vi "UHR-Fleezers Control (fpga) - Leonardo 04-2018 V4.vi"() -> ()   [LabVIEW 2013]
doc: "UHR-Fleezers Instrument Control Code (fpga)"
uses:
  <vilib>/Platform/TimedLoop/XDataNode/timing_clust.ctl
  <vilib>/Platform/TimedLoop/XDataNode/nitl_modes.ctl
  <vilib>/Platform/TimedLoop/XDataNode/wakeup.ctl
  <vilib>/rvi/eio/common/nirviEmuTemplateMethod_errors.vi
  <vilib>/rvi/Emulation/niFpgaSctlEmulationGetInTimedLoop.vi
  <vilib>/rvi/Emulation/niFpgaEmulationReportErrorSimple.vi
  <vilib>/rvi/Emulation/niFpgaGetClockAttributes.vi
  <vilib>/rvi/Emulation/niFpgaCriticalErrorInLSC.vi
  <vilib>/rvi/FIFO/Fifo_Resource/nirvififoEmulationReadFpgaImpl.vi
  <vilib>/rvi/DataTransferAndStorage/Container/Common/niFpgaContainerGetUniqueNameForEmu.vi
  <vilib>/rvi/DataTransferAndStorage/Container/Common/niFpgaContainerExecOnDevCompGetState.vi
  <vilib>/rvi/interface/RandomDataEmulation/nirviRandomDataFPGAFIFO.vi
  <vilib>/rvi/interface/RandomDataEmulation/niFpgaRandomDataHandleErrors.vi
  <vilib>/rvi/eio/common/nirviEmuReportErrorAndStop.vi
  <vilib>/rvi/Emulation/niFpgaProcessEmulError.vi
  <vilib>/rvi/FIFO/Fifo_Resource/nirvififoEmulationWriteFpgaImpl.vi
  <vilib>/Platform/TimedLoop/XDataNode/XDataNode.xnode
  <vilib>/eio/EIOMethodNode/EIOMethodNode.xnode
  <vilib>/eio/EIONode/EIONode.xnode
  <vilib>/rvi/DataTransferAndStorage/Container/XNode/niFpgaContainer.xnode
  <vilib>/rvi/FIFO/Fifo_Resource/nirvififoEmulationRead.vi
  <vilib>/rvi/FIFO/Fifo_Resource/niFpgaFifoEmulationRefIn.vi
  <vilib>/rvi/interface/RandomDataEmulation/nirviRandomDataFpgaReadWriteTemplate.vi
  <vilib>/rvi/FIFO/Fifo_Resource/nirvififoEmulationWrite.vi
  <vilib>/addons/control/pid/fpga.llb/XNode/niFpgaPID.xnode
  <vilib>/Platform/TimedLoop/XDataNode/XDNodeRunTimeDep.lvlib
  <vilib>/rvi/Memory/Memory_Emulation/niFpgaMemoryEmulationRefIn.vi
panel:
  in  "Tab Control 2":T1(tab)
  out "BD1 amplitude 1 out":u16
  out "BD1 amplitude 2 out":u16
  in  "FB output range":cluster{"output low":i16, "output high":i16}={"output low"=0, "output high"=3000}
  in  "FB Gains":T2={"proportional gain (Kc)"=10, "integral gain (Kc*Ts/Ti)"=5, "derivative gain (Kc*Td/Ts)"=0}
  in  "RF synth green feedback max":i16=4000
  in  "RD":bool=TRUE
  in  "Swap F1 and F2":bool
  in  "Scan BD":bool
  in  "Start scan":bool
  in  "OSK Bd 1":bool
  in  "Reset Bd 1":bool
  in  "PMODE":bool=TRUE
  in  "Number Interlace Cycles":u8=2 min=1 max=3
  in  "Interlace Off Parameters":u8=1 min=1 max=3
  in  "Interlace ON/OFF":bool
  out "DIO Relative phase":i16
  in  "Phase count adjustment (DIO)":i16
  in  "+ phase (DIO)":bool
  out "DIO Late Counter":u8
  in  "DIO count 1 (ticks)":u16=400
  in  "DIO count 2 (ticks)":u16=400
  in  "DIO count 3 (ticks)":u16=400
  out "AI2 Y Sum Set 2":i16
  out "AI2 Y Sum Set 1":i16
  in  "FB Setpoint Set 1":i16 min=0 step=1
  in  "FB Reset Set 1":bool
  in  "FB On/Off Set 1":bool
  in  "FB Reset Set 2":bool
  in  "FB On/Off Set 2":bool
  in  "FB Setpoint Set 2":i16 min=0 step=1
  in  "Amp switch delay":u8=5
  in  "RF synth bd controls green":bool
  in  "Phase Trap 2":fxp<+,14,14>
  in  "Phase Trap 1":fxp<+,14,14>
  in  "Phase offset method":u8
  in  "BD 2 Amplitude 1":u16
  in  "BD 1 Amplitude 1":u16
  in  "BD 2 Frequency 1":u64
  in  "BD 1 Frequency 1":u64
  in  "BD 2 Amplitude 2":u16
  in  "BD 1 Amplitude 2":u16
  in  "BD 2 Frequency 2":u64
  in  "BD 1 Frequency 2":u64
  in  "BD 2 Amplitude 3":u16
  in  "BD 1 Amplitude 3":u16
  in  "BD 2 Frequency 3":u64
  in  "BD 1 Frequency 3":u64
  in  "BD 2 Delay (Ticks)":u8 caption="Count(Ticks)"
  in  "Next trap write delay (ticks)":u8 caption="Count(Ticks)"
  out "Random phase generated":fxp<+,14,14>
  in  "RF phase reset before cycles":bool
  in  "Trap 1 osc enable":bool
  in  "N trap osc periods":i16
  in  "Trap osc period (pts)":i16
  in  "Osc traps":bool
  in  "Initiate trap osc":bool
  in  "Ready Write":bool
  in  "Data":i64
  in  "Address 2":u32
  in  "Osc trap cont.":bool
  in  "Trap 2 osc enable":bool
  out "green FB running":bool
  in  "APD 2 AO scale factor":i16=1
  in  "BD 1 Delay (ticks)":u8
  in  "Tab Control":T3(tab)=enum."MCL trap control"
  in  "Set 3":bool
  in  "Set 2":bool=TRUE
  in  "Set 1":bool=TRUE
  in  "Trap Pos to FIFO":bool
  in  "N of AI1 Int Acq Sets":i16=2 min=1 max=3 step=1
  out "AI Late Counter":u8
  in  "ai count":u16=400
  in  "+ phase":bool
  in  "Phase count adjustment":i16
  out "Relative phase":i16
  in  "AI to FIFO":bool
  out "BD1 Frequency Out 1":u64
  out "BD1 Frequency Out 2":u64
  out "Trap Pos FIFO Timeout":u16
  out "Trap AI FIFO Timeout":u16
  in  "Trap FIFO Set Timeout":i32
  in  "Scan freq.  increment":i64
  in  "Scan steps":u64
  in  "Number of scans":u16
  in  "Cycles per step":u64
  in  "Raster setpoint":fxp<+/-,16,1>
  in  "Raster to target force":bool
  out "Actual Scan freq":u64
  in  "Cont. Scan":bool
  out "Scan I":u64
  in  "Abort scan":bool
  out "Scanning":bool
  in  "FB Min frequency":u64
  in  "FB Max Frequency":u64
  in  "Dynamic Force FB (Ronen)":bool
  in  "Trap pos. FB Range":T4={"FB2 output low"=-1.0, "FB2 output high"=0.999969482421875}
  in  "Trap Pos. FB Gains":T5={"proportional gain (Kc)"=0.999969482421875, "integral gain (Kc*Ts/Ti)"=0.999969482421875, "derivative gain (Kc*Td/Ts)"=0.0}
  in  "B factor":fxp<+/-,32,16>
  in  "Negate Diff?":bool
  in  "Diff FB Measurement?":bool
  in  "FB Trig Integrate":u32=1
  out "TTrig?":bool
  in  "TTrig Negate Pos":bool=TRUE
  out "Trap Pos FB Int Signal":fxp<+/-,24,9> format="%.18g"
  out "Trap Pos FB Int-Norm Signal":fxp<+/-,16,1> format="%.16g"
  in  "FPGA TTrig Thresh":i64
  in  "FPGA Trap Trig":bool
  out "Trap Pos FB Action":i64
  in  "Trap Pos. FB Offset Factor":i64
  in  "Trap Pos. FB Mult Factor":i64=2
  in  "Trap Pos. FB Reset":bool
  in  "Trap Pos FB Monitor T1 or T2":bool
  in  "AI1 X Scale":u16
  in  "Trap Pos FB Int Count":u16=100
  in  "Trap Pos FB Negate Action":bool
  out "AI1 X Set 2":fxp<+/-,16,1>
  out "AI1 X Set 1":fxp<+/-,16,1>
  in  "Trap Pos. FB SP":fxp<+/-,16,1>
  in  "Force feedback":bool
  out "TTrig Sig":i64
  out "TTrig Fin Thresh":i64
  in  "1D or 2D Scan?":bool
  in  "Abort scan (MCL)":bool
  in  "MCL Scan Axis":bool
  in  "Cont. Scan (MCL)":bool
  out "Scan I (MCL)":u64
  in  "Number of scans (MCL)":u16
  out "Scanning MCL":bool
  in  "Scan steps (MCL)":u64
  in  "Cycles per step (MCL)":u64
  in  "Scan freq.  increment (MCL)":i16
  in  "Start scan (MCL)":bool
  in  "AO2 (X)":i16
  in  "AO1 (Y)":i16
  out "MCL Late Counter":u8
  in  "MCL count":u32=800
  out "MCL Relative Phase":i16
  in  "Phase count adjustment (MCL)":i16
  in  "+ phase (MCL)":bool
  in  "Lifetime events to read blue":u16=100
  in  "Lifetime read blue fifo":bool
  out "lifetime events in fifo":u16
  out "APD2 int gate":bool
  in  "APD Gate Operating Mode":u8 max=2 step=1
  in  "Invert APD Gate":bool
  in  "APD Gate OFF Count":u16=100
  in  "APD Gate ON Count":u16=300
  out "APD 1 Gate Late Counter":u8
  out "APD 1 Gate Relative Phase":i16
  in  "Phase count adjustment (APD 1 Gate)":i16
  in  "+ phase (APD 1 Gate)":bool
  out "APD 2 Counts 0":u32
  out "APD 2 Counts 1":u32
  out "APD 1 Counts 0":u32
  out "APD 1 Counts 1":u32
  in  "Phase count adjustment (APD 2 Gate)":i16
  out "APD 2 Gate Late Counter":u8
  out "APD 2 Gate Relative Phase":i16
  in  "+ phase (APD 2 Gate)":bool
  out "APD 3 Counts 0":u32
  out "APD 3 Counts 1":u32
  out "APD 3 Gate Late Counter":u8
  in  "Phase count adjustment (APD 3 Gate)":i16
  out "APD 3 Gate Relative Phase":i16
  in  "+ phase (APD 3 Gate)":bool
  out "APD1 int gate":bool
  out "APD3 int gate":bool
  in  "Lifetime timeout APD1":u16=200
  in  "APD to FIFO":bool
  in  "APD Acq Rate Count":u32=20000000
  out "APD Acq Late Counter":u16
  out "APD Acq Relative Phase":i16
  in  "+ phase (APD Acq)":bool
  in  "Phase Count Adjustment (APD Acq)":i16
  in  "APD 1 AO scale factor":i16=1
  out "APD2 out state":bool
  out "APD1 out state":bool
  out "APD Acq Late?":bool
  in  "Number of OFF cycles":i16
  in  "Green long-scale interlacing":bool
  in  "D3 2":i16
  in  "I3 2":i16=5
  in  "P3 2":i16=10
  in  "Green FB Setpoint 2":i16=250 min=0 step=1
  in  "Green FB Reset 2":bool
  in  "Green Filter Flipper":bool
  in  "Green interlace OFF count":u16=100
  out "GI Relative phase":i16
  in  "Phase count adjustment (GI)":i16
  in  "+ phase (GI)":bool
  in  "Green interlace ON count":u16=300
  out "GI Late Counter":u8
  in  "Invert GI":bool
  in  "Operating Mode":u8 max=2 step=1
  in  "Current Out":u16=30000
  in  "Green int current ON count adj":u32=150
  in  "Green interlace OFF count 2":u32=900
  in  "Green interlace ON count 2":u32=300
  out "GI Late Counter 2":u16
  in  "Green FB Count":u32=1200
  in  "Phase count adjustment (GI) 2":i16=20
  in  "Green FB Setpoint":i16=250 min=0 step=1
  in  "Invert GI 2":bool
  out "GI Relative phase 2":i16
  in  "+ phase (GI) 2":bool
  in  "Phase count adjustment (Green FB)":i16=10
  out "Green Late Counter":u16
  out "Green FB Relative Phase":i16
  in  "+ phase (Green FB)":bool
  out "Green FB Signals":T6
  out "Green FB Sum":i16
  in  "Green FB Gains":T2={"proportional gain (Kc)"=10, "integral gain (Kc*Ts/Ti)"=5, "derivative gain (Kc*Td/Ts)"=0}
  in  "Green FB On/Off":bool
  in  "Green FB Reset":bool
  out "Green FB Late?":bool
  out "GI Late?":bool
  in  "Operating Mode 2":u8=2 max=2 step=1
  in  "Chassis2/Mod4/AO1":u16
  in  "Number of ON cycles":i16
  in  "+ phase (RI)":bool
  out "RI Relative phase":i16
  out "RI Late Counter":u8
  in  "Red interlace ON count":u16=300
  in  "Red interlace OFF count":u16=100
  in  "Invert RI":bool
  in  "Red Laser Operating Mode":u8 max=2 step=1
  in  "Phase count adjustment (RI)":i16
  in  "Phase count adjustment (BI D)":i16
  in  "Blue Laser Operating Mode (D)":u8 max=2 step=1
  in  "Invert BI (D)":bool
  in  "Blue interlace OFF count (D)":u16=100
  in  "Blue interlace ON count (D)":u16=300
  out "Blue Late Counter (D)":u8
  out "BI Relative phase (D)":i16
  in  "+ phase (BI D)":bool
  in  "Lifetime to FIFO":bool
  out "lifetime (ticks)":u16
  # "Raster Scan AOD"
  # "1 (X)"
  # "2 (Y)"
  # "IR Intensity Feedback (RF BD 1)"
  # "FB Gains Set 1"
  # "FB output range 1"
  # "IR Intensity Feedback (RF BD 2) -\nonly when using BD 2 for green laser AOM (not trap Y)"
  # "Keep below 4096 (12 bits) to stay within range of RF board. Going over doesn't saturate, it truncates higher bits."
  # "RF phase offset control"
  # "Methods are:\n0 - Default, do nothing at all (no phase offset writes)\n1 - Manual phase adjustment\n2 - Cycle the phase adjustment using the input phase numbers as increment values for each cycle"
  # "False is usual, True is external loop method"
  # "Parameters if using the external RF switching loop"
  # "Parameters if using the usual internal RF switching method"
  # "FB Triggering Excitation Laser"
  # "Trap Pos. FB Gains"
  # "Trap Pos. FB Range"
  # "AO1 (Y)"
  # "2D"
  # "Trap 3"
  # "1D"
  # "AO2 (X)"
  # "Fl Laser"
  # "APD AO for aligning"
  # "Detection Loop"
  # "Green fluorescent laser digital gate interlacing loop"
  # "0 Forced ON\n1 Forced OFF\n2 Interlacing"
  # "ALEX settings:"
  # "Controls for usual IA ME controls green AOM"
  # "Controls for RF synth board controls green AOM"
  # "Green FB Gains"
  # "Red fluorescent laser digital gate interlacing loop"
  # "Detection Loop"
  # "0 Forced ON\n1 Forced OFF\n2 Interlacing"
  # "Analog/FB Control Loop\n(Disabled)"
  # "Digital Control Loop"
  # "Blue laser intensity reading"
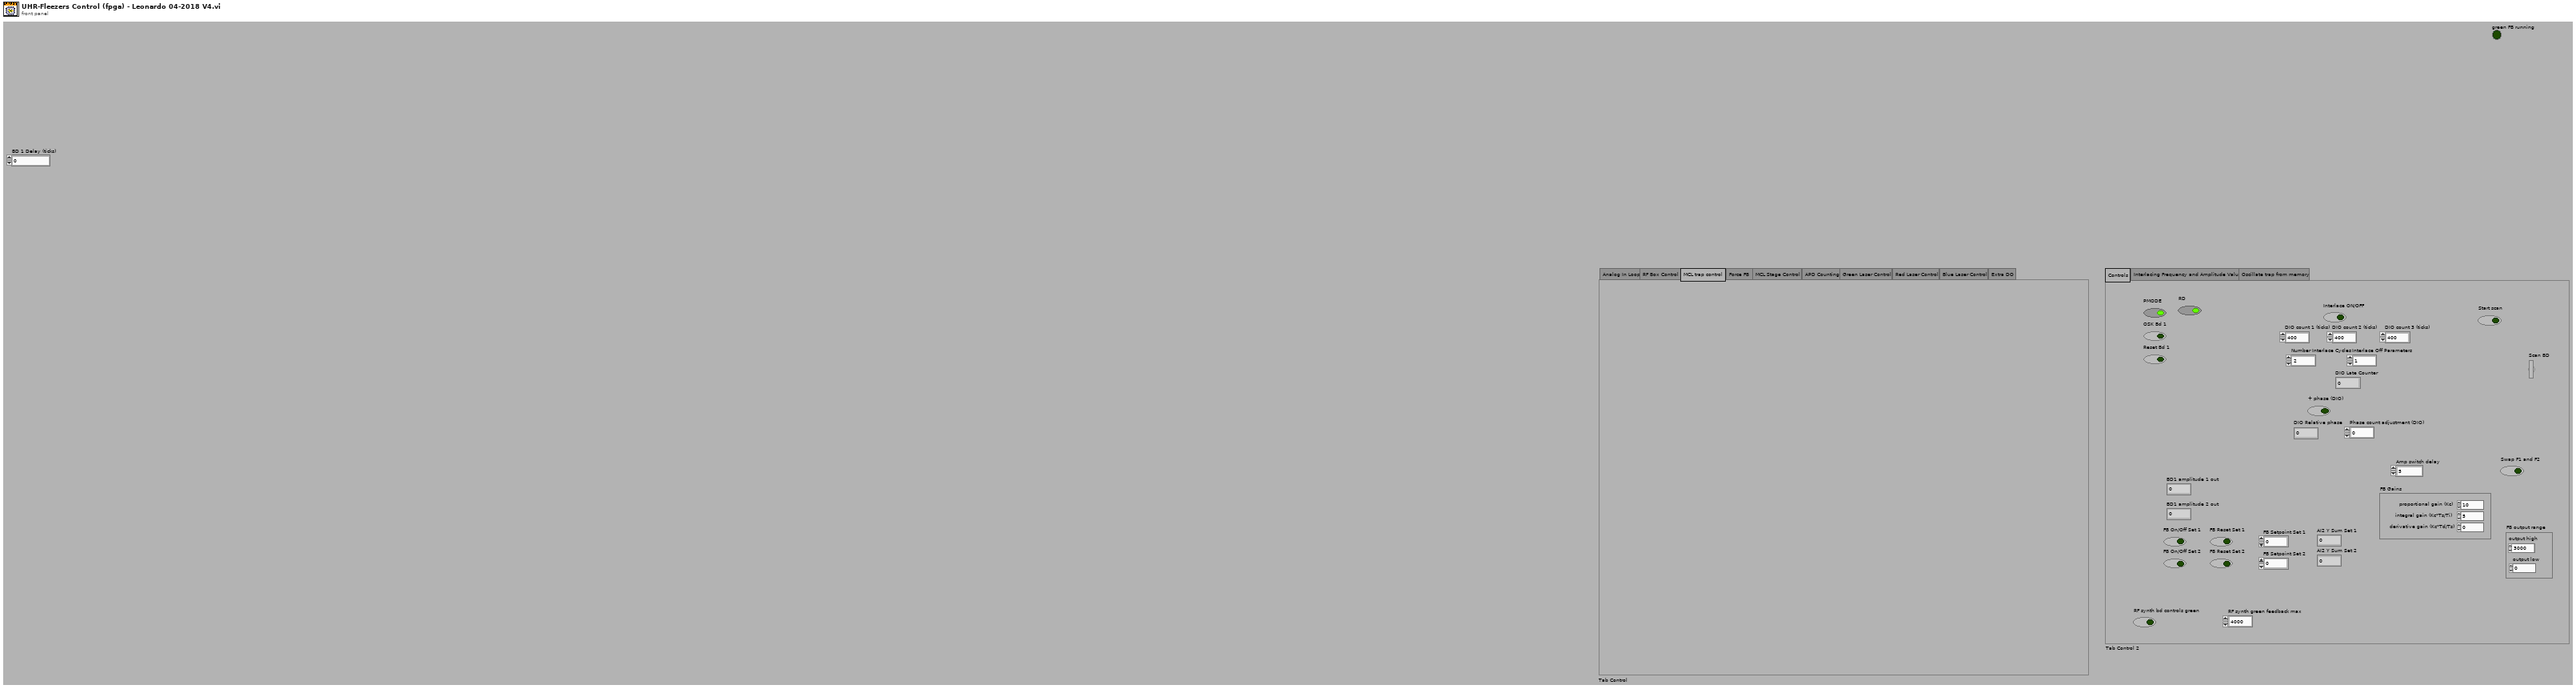
[diagram p1: front panel]
types:
  T1 = enum32{"Controls", "Interlacing Frequency and Amplitude Values", "Oscillate trap from memory"}
  T2 = cluster{"proportional gain (Kc)":i16, "integral gain (Kc*Ts/Ti)":i16, "derivative gain (Kc*Td/Ts)":i16}
  T3 = enum32{"Analog In Loop", "RF Box Control", "MCL trap control", "Force FB", "MCL Stage Control", "APD Counting", "Green Laser Control", "Red Laser Control", "Blue Laser Control", "Extra DO"}
  T4 = cluster{"FB2 output low":fxp<+/-,16,1>, "FB2 output high":fxp<+/-,16,1>}
  T5 = cluster{"proportional gain (Kc)":fxp<+/-,16,1>, "integral gain (Kc*Ts/Ti)":fxp<+/-,16,1>, "derivative gain (Kc*Td/Ts)":fxp<+/-,16,1>}
  T6 = cluster{"Green FB Ch 0":i16, "Green FB Ch 1":i16, "Green FB Ch 2":i16}
  T7 = typedef "XDNodeRunTimeDep.lvlib/timing_clust.ctl" = cluster{"Expected End [f-1]":u64, "Actual End [f-1]":u64, "Finished Late? [f-1]":bool, "Expected End [i-1]":u64, "Actual End [i-1]":u64, "Finished Late? [i-1]":bool, "Expected Start [i]":u64, "Actual Start [i]":u64, "Expected Start [f]":u64, "Actual Start [f]":u64, "Source Name":string, "Structure Name":string, "Period":i64, "Deadline":i64, "Offset":i64, "Start":i64, "Priority":i32, "Timeout":i32, "Mode":T8, "Wakeup Reason":T9, "Error":errorcluster, "Source Type":string, "Secondary Source Type":string, "Global End Time":u64, "Global Start Time":u64, "Frame Duration":u64, "Iteration Duration":u64, "Assigned CPU":i32, "I/O Scan Engine Mode":u32}
  T8 = typedef "XDNodeRunTimeDep.lvlib/nitl_modes.ctl" = enum32{"No Change", "Process missed periods, maintain original phase", "Discard missed periods, maintain original phase", "Process missed periods, ignore original phase", "Discard missed periods, ignore original phase"}
  T9 = typedef "XDNodeRunTimeDep.lvlib/wakeup.ctl" = enum32{"Normal", "Aborted", "Asynchronous wakeup", "Timing source error", "Timed loop error", "Timeout"}
  T10 = cluster{"Chassis2/Mod2/AI0":i16, "Chassis2/Mod2/AI1":i16, "Chassis2/Mod2/AI2":i16}
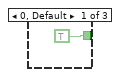
[diagram p2: hidden frame]
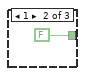
[diagram p3: hidden frame]
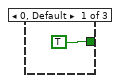
[diagram p6: hidden frame]
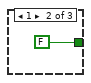
[diagram p7: hidden frame]
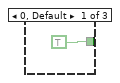
[diagram p11: hidden frame]
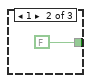
[diagram p12: hidden frame]
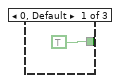
[diagram p13: hidden frame]
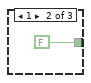
[diagram p14: hidden frame]
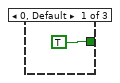
[diagram p18: hidden frame]
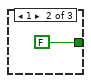
[diagram p19: hidden frame]
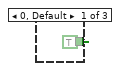
[diagram p20: hidden frame]
diagram:
  w3 = FALSE
  w4 = FALSE
  # "BD2 amp"
  # "BD1 amp"
  # "BD2 amp"
  # "BD1 amp"
  # "timing array current index"
  # "timing array"
  # "timing counter (phase adjusted here)"
  # "late counter"
  n1 = while {
    stop <- FALSE stop-if-true
    n2 = xnode "FPGA I/O Node"("Connector0/DIO3"="Green Filter Flipper", "Chassis2/Mod1/AO1"="Chassis2/Mod4/AO1") -> ()  [unwired: 2 in, 2 out]
    n3 = call "Loop Timer11"("Count(Ticks)"=u32 40000 ("Extra DO Counts")) -> ()  [unwired: 1 out]
  }
  n4 = disable-structure shown="Disabled" {
    frame Disabled {
      w18 = i16 2 items=["UnSet Ready", "ReadWrite", "Wait Ready"]
      n5 = while "Handshake memory transfer for trap oscillation sin wave data" {
        shift-right: [w20] -> _
        shift-left: w18 -> [w21]
        stop <- FALSE stop-if-true
        # "Write"
        n6 = case shown="1" w21 {
          tunnel: [w24 w29 w30] -> w20
          frame 3, Default {
            w22 = i16 2 items=["UnSet Ready", "ReadWrite", "Wait Ready"]
            w23 = i16 1 items=["UnSet Ready", "ReadWrite", "Wait Ready"]
            n7 = Select(t=w23, s="Ready Write", f=w22) -> (s? t:f=w24:i16)
          }
          frame 1 {
            w29 = i16 0 items=["UnSet Ready", "ReadWrite", "Wait Ready"]
            n8 = xnode ("Memory Write")("Address"="Address 2", "Data"="Data", "Memory In"=refnum<k21> "Trap osc memory") -> ()  [unwired: 1 out]
          }
          frame 0 {
            w30 = i16 2 items=["UnSet Ready", "ReadWrite", "Wait Ready"]
            n9 = local write "Ready Write"(FALSE ("Ready Read")) -> ()
          }
        }
      }
    }
    frame Enabled {
    }
  }
  n10 = flat-sequence "FPGA initialization to do before running any of the loops" {
    tunnel: [u16 0 ("DIO count 3 (ticks)")] -> w2
    tunnel: [w39] -> _
    frame #0 {
      # "UDCLK out enable and set low"
      # "WR"
      # "BD 2"
      # "BD 1"
      # "With the RF synth board initialization now done in a separate fpga vi, now when this vi is started, board is already configured and is ready for interlacing. Just need to set WR high and enabled UDCLK as write and set to low.\nbefore setting data and address bits."
      # "Start up expansion chassis early\nto avoid delays later"
      # "Set data and address values to something safe (a correct setting) so any initial WR and udclk flipping doesn't have a chance to mess anything up. Safe would be setting an unused data entry:"
      n11 = xnode "FPGA I/O Method Node"("Enable"=TRUE) -> ("FPGA I/O Out"=w33:refnum<k21>)  [unwired: 1 in]
      n12 = xnode "FPGA I/O Method Node"("Enable"=TRUE) -> ("FPGA I/O Out"=w36:refnum<k21>)  [unwired: 1 in]
      n13 = xnode "FPGA I/O Node"("Chassis2/Mod1/AO0"=u16 0 ("Chassis2/Mod4/AO0")) -> ("Chassis2/Mod2/AI0"=w39:i16)  [unwired: 2 in, 2 out]
      n14 = xnode "FPGA I/O Node"("Connector1/DIO15"=TRUE) -> ()  [unwired: 1 in, 1 out]
      n15 = xnode "FPGA I/O Node"("I/O Item"=FALSE ("Connector1/DIO30"), "FPGA I/O In"=w33) -> ()  [unwired: 1 out]
      n16 = xnode "FPGA I/O Node"("I/O Item"=FALSE ("Connector1/DIO30"), "FPGA I/O In"=w36) -> ()  [unwired: 1 out]
      n17 = xnode "FPGA I/O Node"("Connector1/DIO0"=FALSE, "Connector1/DIO1"=FALSE, "Connector1/DIO2"=FALSE, "Connector1/DIO3"=FALSE, "Connector1/DIO4"=FALSE, "Connector1/DIO5"=FALSE, "Connector1/DIO6"=FALSE, "Connector1/DIO7"=FALSE, "Connector1/DIO8"=FALSE, "Connector1/DIO9"=FALSE, "Connector1/DIO10"=FALSE, "Connector1/DIO11"=FALSE, "Connector1/DIO12"=FALSE, "Connector1/DIO13"=FALSE, "Connector1/DIO20"=FALSE, "Connector1/DIO21"=FALSE, "Connector1/DIO22"=FALSE, "Connector1/DIO23"=FALSE, "Connector1/DIO24"=FALSE, "Connector1/DIO25"=FALSE, "Connector1/DIO26"=FALSE, "Connector1/DIO27"=FALSE, "Connector1/DIO14"=FALSE) -> ()  [unwired: 23 in, 23 out]
    }
  }
  n18 = node-c288() -> (w10:T7)  [unwired: 1 in]
  n19 = timed-loop "RF box board DIO control: control bits" {
    timing: w10 -> [_]
    timing-out: [_] -> w9
    tunnel: [w66] -> _
    tunnel: w2 -> [w66]
    stop <- FALSE stop-if-true
    n20 = xnode "FPGA I/O Node"("Connector1/DIO16"="RD", "Connector1/DIO17"="PMODE", "Connector1/DIO18"="OSK Bd 1", "Connector1/DIO19"="Reset Bd 1") -> ()  [unwired: 4 in, 4 out]
  }
  n21 = node-c288(w9) -> ()
  n22 = local read "AO1 (Y)"() -> (w12:i16)
  n23 = local read "AO2 (X)"() -> (w11:i16)
  n24 = To Unsigned Long Integer(number=w2) -> (unsigned 32bit integer=w5:u32)
  n25 = disable-structure shown="Disabled" {
    disable-tunnel: w4 -> [w74 _]
    disable-tunnel: w2 -> [w73 _]
    frame Disabled {
      n26 = while "APD 2 Gating" {
        shift-right: [w78] -> _
        shift-left: w73 -> [w83]
        shift-right: [w77] -> _
        shift-left: w74 -> [w75]
        stop <- FALSE stop-if-true
        n27 = flat-sequence {
          tunnel: w83 -> [w86]
          tunnel: [w87] -> w81
          tunnel: [w86] -> w79
          tunnel: [w85] -> w76
          tunnel: w75 -> [w85]
          tunnel: [w90] -> w82
          tunnel: w81 -> [w90]
          tunnel: [w89] -> w80
          tunnel: w79 -> [w89]
          tunnel: w76 -> [w88]
          tunnel: [w112] -> w78
          tunnel: w82 -> [w122]
          tunnel: w80 -> [w120]
          tunnel: [w91] -> w77
          frame #0 {
            n28 = call "Loop Timer3"("Count(Ticks)"=w86) -> ("Tick Count(Ticks)"=w87:u32)
          }
          frame #1 {
            # "Signal maybe then sent through \na transistor before APD"
            n29 = xnode "FPGA I/O Node"("Connector1/DIO34"=w88) -> ()  [unwired: 1 in, 1 out]
            "APD2 int gate" <- w88
          }
          frame #2 {
            n30 = local read "APD Gate ON Count"() -> (w105:u16)
            n31 = local read "APD Gate OFF Count"() -> (w104:u16)
            n32 = feedback #1(TRUE) -> (w117:bool)
            n33 = feedback-in #2(w122) -> ()
            n34 = feedback #2(w122) -> (w106:u32)
            n35 = Not(x=w117) -> (.not. x?=w115:bool)
            n36 = feedback-in #1(w115) -> ()
            n37 = Subtract(x=w122, y=w106) -> (x-y=w121:u32)
            n38 = Select(t=w105, s=w115, f=w104) -> (s? t:f=w119:u16)
            n39 = Subtract(x=w121, y=w120) -> (x-y=w97:u32)
            n40 = Subtract(x=w119, y=w97) -> (x-y=w111:u32)
            n41 = Number To Boolean Array(number=w97) -> (Boolean array=w96:bool[])
            n42 = Or Array Elements(Boolean array=w96) -> (logical OR=w95:bool)
            n43 = Boolean To (0,1)(Boolean="+ phase (APD 2 Gate)") -> (0, 1=w109:i16)
            n44 = Multiply(x=w109, y="Phase count adjustment (APD 2 Gate)") -> (x*y=w107:i16)
            n45 = Boolean To (0,1)(Boolean=w95) -> (0, 1=w102:i16)
            n46 = Add(x=w111, y=w107) -> (x+y=w112:u32)
            n47 = To Unsigned Byte Integer(number=w102) -> (unsigned 8bit integer=w99:u8)
            n48 = feedback #3(i16 0) -> (w114:i16)
            n49 = Subtract(x=w114, y=w107) -> (x-y=w113:i16)
            "APD 2 Gate Relative Phase" <- w113
            n50 = feedback-in #3(w113) -> ()
            n51 = feedback #4(u8 0) -> (w100:u8)
            n52 = Add(x=w99, y=w100) -> (x+y=w98:u8)
            "APD 2 Gate Late Counter" <- w98
            n53 = feedback-in #4(w98) -> ()
            n54 = local read "APD Gate Operating Mode"() -> (w103:u8)
            n55 = case shown="2" w103 {
              tunnel: [TRUE FALSE w125] -> w92
              tunnel: w117 -> [_ _ w125]
              frame 0, Default {
              }
              frame 1 {
              }
              frame 2 {
              }
            }
            n56 = local read "Invert APD Gate"() -> (w94:bool)
            n57 = Not(x=w92) -> (.not. x?=w93:bool)
            n58 = Select(t=w93, s=w94, f=w92) -> (s? t:f=w91:bool)
          }
        }
      }
    }
    frame Enabled {
    }
  }
  n59 = while "DAQ AI set 1" {
    shift-right: [w126] -> _
    shift-left: w2 -> [w131]
    stop <- FALSE stop-if-true
    n60 = flat-sequence {
      tunnel: w131 -> [w142]
      tunnel: [w141] -> w129
      tunnel: [w142] -> w128
      tunnel: [w152] -> w139
      tunnel: [w151] -> w138
      tunnel: [w150] -> w137
      tunnel: [w149] -> w136
      tunnel: [w148] -> w135
      tunnel: [w147] -> w134
      tunnel: [w146] -> w133
      tunnel: [w145] -> w132
      tunnel: [w144] -> w130
      tunnel: w129 -> [w144]
      tunnel: w128 -> [w143]
      tunnel: [w143] -> w127
      tunnel: [w182] -> w126
      tunnel: w139 -> [w208]
      tunnel: w138 -> [w174]
      tunnel: w137 -> [w175]
      tunnel: w136 -> [w154]
      tunnel: w135 -> [w198]
      tunnel: w134 -> [w197]
      tunnel: w133 -> [w196]
      tunnel: w132 -> [w195]
      tunnel: w130 -> [w192]
      tunnel: w127 -> [w189]
      frame #0 {
        n61 = call "Loop Timer"("Count(Ticks)"=w142) -> ("Tick Count(Ticks)"=w141:u32)
      }
      frame #1 {
        n62 = xnode "FPGA I/O Node"("Connector1/DIO31"=TRUE ("Connector1/DIO33")) -> ("Connector0/AI0"=w152:i16, "Connector0/AI1"=w151:i16, "Connector0/AI2"=w150:i16, "Connector0/AI3"=w149:i16, "Connector0/AI4"=w148:i16, "Connector0/AI5"=w147:i16, "Connector0/AI6"=w146:i16, "Connector0/AI7"=w145:i16)  [unwired: 9 in, 9 out]
      }
      frame #2 {
        w178 = FALSE ("AI to FIFO")
        # "Normalize by trap bead QPD sum, AI3"
        # "Adjust phase after data acquired if button pressed"
        n63 = feedback #5(i16 1) -> (w201:i16)
        n64 = Increment(x=w201) -> (x+1=w207:i16)
        n65 = Scale By Power Of 2(n="AI1 X Scale", x=w174) -> (x*2^n=w172:i16)
        n66 = Greater?(x=w207, y="N of AI1 Int Acq Sets") -> (0:w204:bool)
        n67 = Select(t=i16 1, s=w204, f=w207) -> (s? t:f=w206:i16)
        n68 = feedback-in #5(w206) -> ()
        n69 = Divide(x=w172, y=w154) -> (x/y=w171:fxp<+/-,16,1>)
        n70 = feedback #6(w178) -> (w176:bool)
        n71 = feedback #7(w178) -> (w194:bool)
        n72 = case shown="1, Default" w201 {
          tunnel: w175 -> [w231 w238 _]
          tunnel: ["Set 1" "Set 2" "Set 3"] -> w199
          tunnel: ["AI to FIFO" w240 w245] -> w193
          tunnel: w194 -> [_ w240 w245]
          tunnel: ["Trap Pos to FIFO" w239 w244] -> w177
          tunnel: w176 -> [_ w239 w244]
          tunnel: w171 -> [w230 w237 _]
          tunnel: [w229 w235 FALSE] -> w158
          tunnel: [w228 w236 u64 0 ("BD1 Frequency Out 2")] -> w157
          frame 1, Default {
            n73 = local read "BD1 Frequency Out 1"() -> (w228:u64)
            n74 = Compound Arithmetic op=AND("Trap Pos to FIFO", "Set 1", "AI to FIFO") -> (w229:bool)
            "AI2 Y Sum Set 1" <- w231
            "AI1 X Set 1" <- w230
          }
          frame 2 {
            n75 = local read "BD1 Frequency Out 2"() -> (w236:u64)
            n76 = Compound Arithmetic op=AND(w239, "Set 2", w240) -> (w235:bool)
            "AI2 Y Sum Set 2" <- w238
            "AI1 X Set 2" <- w237
          }
          frame 3 {
          }
        }
        n77 = And(x=w199, y=w193) -> (x .and. y?=w200:bool)
        n78 = case shown="True" w200 {
          tunnel: w208 -> [_ w259]
          tunnel: w174 -> [_ w258]
          tunnel: w175 -> [_ w257]
          tunnel: w154 -> [_ w256]
          tunnel: w198 -> [_ w255]
          tunnel: w197 -> [_ w254]
          tunnel: w196 -> [_ w253]
          tunnel: w195 -> [_ w252]
          tunnel: 0 ("DMA buffer timeout") -> [_ w261]
          frame False {
          }
          frame True {
            n79 = Build Array(w259, w258, w257, w256, w255, w254, w253, w252) -> (w260:i16[])
            n80 = for {
              tunnel: w260 -> [w263] mode=indexing
              tunnel: w261 -> [w264]
              tunnel: [w262] -> w250 mode=indexing
              n81 = xnode ("FIFO Write")("Element"=w263, "Timeout"=w264) -> ("Timed Out?"=w262:bool)  [unwired: 1 in, 1 out]
            }
            n82 = Or Array Elements(Boolean array=w250) -> (logical OR=w247:bool)
            n83 = Boolean To (0,1)(Boolean=w247) -> (0, 1=w249:i16)
            n84 = feedback #8(u16 0) -> (w248:u16)
            n85 = Add(x=w249, y=w248) -> (x+y=w246:u16)
            "Trap AI FIFO Timeout" <- w246
            n86 = feedback-in #8(w246) -> ()
          }
        }
        n87 = feedback-in #6(w177) -> ()
        n88 = feedback-in #7(w193) -> ()
        n89 = case shown="True" w158 {
          tunnel: w157 -> [_ w214]
          tunnel: [u8 0 w211] -> w156
          frame False {
          }
          frame True {
            n90 = Split Number(x=w214) -> (hi(x)=w215:u32, lo(x)=w216:u32)
            n91 = Split Number(x=w215) -> (lo(x)=w217:u16)  [unwired: 1 out]
            n92 = Split Number(x=w216) -> (hi(x)=w218:u16, lo(x)=w219:u16)
            n93 = Build Array "BD 1 nu Stack"(w217, w218, w219) -> (w213:u16[])
            n94 = for {
              tunnel: w213 -> [w226] mode=indexing
              shift-right: [w222] -> w211
              shift-left: u8 0 -> [w223]
              n95 = xnode ("FIFO Method Node")("Element"=w226, "Timeout"="Trap FIFO Set Timeout") -> ("Timed Out?"=w225:bool)  [unwired: 1 in, 1 out]
              n96 = Boolean To (0,1)(Boolean=w225) -> (0, 1=w224:i16)
              n97 = To Unsigned Byte Integer(number=w224) -> (unsigned 8bit integer=w221:u8)
              n98 = Add(x=w221, y=w223) -> (x+y=w222:u8)
            }
          }
        }
        n99 = To Unsigned Word Integer(number=w156) -> (unsigned 16bit integer=w155:u16)
        n100 = feedback #9(u16 0) -> (w169:u16)
        n101 = Add(x=w155, y=w169) -> (x+y=w168:u16)
        "Trap Pos FIFO Timeout" <- w168
        n102 = feedback-in #9(w168) -> ()
        n103 = feedback-in #10(w192) -> ()
        n104 = feedback #10(w192) -> (w191:u32)
        n105 = Subtract(x=w192, y=w191) -> (x-y=w190:u32)
        n106 = xnode "FPGA I/O Node"("Connector1/DIO31"=FALSE ("Connector1/DIO34")) -> ()  [unwired: 1 in, 1 out]
        n107 = Subtract(x=w190, y=w189) -> (x-y=w160:u32)
        n108 = Boolean To (0,1)(Boolean="+ phase") -> (0, 1=w185:i16)
        n109 = Multiply(x=w185, y="Phase count adjustment") -> (x*y=w179:i16)
        n110 = Subtract(x="ai count", y=w160) -> (x-y=w183:u32)
        n111 = Number To Boolean Array(number=w160) -> (Boolean array=w161:bool[])
        n112 = feedback #11(i16 0) -> (w181:i16)
        n113 = Add(x=w183, y=w179) -> (x+y=w182:u32)
        n114 = Subtract(x=w181, y=w179) -> (x-y=w180:i16)
        "Relative phase" <- w180
        n115 = feedback-in #11(w180) -> ()
        n116 = Or Array Elements(Boolean array=w161) -> (logical OR=w159:bool)
        n117 = Boolean To (0,1)(Boolean=w159) -> (0, 1=w166:i16)
        n118 = To Unsigned Byte Integer(number=w166) -> (unsigned 8bit integer=w163:u8)
        n119 = feedback #12(u8 0) -> (w164:u8)
        n120 = Add(x=w163, y=w164) -> (x+y=w162:u8)
        "AI Late Counter" <- w162
        n121 = feedback-in #12(w162) -> ()
      }
    }
  }
  n122 = while "MCL stage control" {
    shift-right: [w277] -> _
    shift-left: w2 -> [w280]
    shift-right: [w270] -> _
    shift-left: w12 -> [w267]
    shift-right: [w269] -> _
    shift-left: w11 -> [w265]
    stop <- FALSE stop-if-true
    n123 = flat-sequence {
      tunnel: w280 -> [w283]
      tunnel: [w282] -> w276
      tunnel: [w283] -> w274
      tunnel: [w285] -> w268
      tunnel: w267 -> [w285]
      tunnel: [w284] -> w266
      tunnel: w265 -> [w284]
      tunnel: w276 -> [w289]
      tunnel: [w289] -> w275
      tunnel: w274 -> [w288]
      tunnel: [w288] -> w273
      tunnel: w268 -> [w287]
      tunnel: w266 -> [w286]
      tunnel: w275 -> [w297]
      tunnel: w273 -> [w296]
      tunnel: [w297] -> w279
      tunnel: [w296] -> w278
      tunnel: [w295] -> w272
      tunnel: [w294] -> w271
      tunnel: [w369] -> w277
      tunnel: w279 -> [w376]
      tunnel: w278 -> [w373]
      tunnel: w272 -> [w371]
      tunnel: w271 -> [w370]
      tunnel: [w371] -> w270
      tunnel: [w370] -> w269
      frame #0 {
        n124 = call "Loop Timer3"("Count(Ticks)"=w283) -> ("Tick Count(Ticks)"=w282:u32)
      }
      frame #1 {
        n125 = xnode "FPGA I/O Node"("Connector0/AO1"=w287, "Connector0/AO2"=w286) -> ()  [unwired: 2 in, 2 out]
      }
      frame #2 {
        n126 = local read "Scanning MCL"() -> (w309:bool)
        n127 = Or(x=w309, y="Start scan (MCL)") -> (x .or. y?=w304:bool)
        n128 = Not(x="Abort scan (MCL)") -> (.not. x?=w302:bool)
        n129 = And(x=w302, y=w304) -> (x .and. y?=w301:bool)
        n130 = case "Raster scan" shown="False" w301 {
          tunnel: [w310 w353] -> w306
          tunnel: "Start scan (MCL)" -> [_ w338]
          tunnel: [w310 w314] -> w290
          frame False {
            w310 = i16 0
            n131 = local write "Scanning MCL"(FALSE ("scanning")) -> ()
          }
          frame True {
            w324 = i16 0
            w323 = u64 0
            # "scan incr."
            # "freq. incr. mult."
            # "count steps"
            # "count number of cycles"
            n132 = feedback #13(w323) -> (w350:u64)
            n133 = Select(t=w323, s=w338, f=w350) -> (s? t:f=w352:u64)
            n134 = Increment(x=w352) -> (x+1=w349:u64)
            n135 = Greater?(x="Cycles per step (MCL)", y=w349) -> (0:w333:bool)
            n136 = Select(t=w349, s=w333, f=w323) -> (s? t:f=w348:u64)
            n137 = feedback-in #13(w348) -> ()
            n138 = feedback #14(w323) -> (w347:u64)
            n139 = Select(t=w323, s=w338, f=w347) -> (s? t:f=w342:u64)
            n140 = Increment(x=w342) -> (x+1=w346:u64)
            n141 = Add(x="Scan steps (MCL)", y="Scan steps (MCL)") -> (x+y=w345:u64)
            n142 = Select(t=w342, s=w333, f=w346) -> (s? t:f=w328:u64)
            n143 = Greater?(x=w345, y=w328) -> (0:w327:bool)
            n144 = Select(t=w328, s=w327, f=w323) -> (s? t:f=w343:u64)
            n145 = feedback-in #14(w343) -> ()
            n146 = Equal?(x="Scan steps (MCL)", y=w328) -> (x = y?=w332:bool)
            n147 = Greater?(x="Scan steps (MCL)", y=w342) -> (0:w341:bool)
            n148 = feedback #15(w324) -> (w344:i16)
            n149 = Select(t=w324, s=w338, f=w344) -> (s? t:f=w330:i16)
            n150 = Increment(x=w330) -> (x+1=w340:i16)
            n151 = Decrement(x=w330) -> (x-1=w339:i16)
            n152 = Select(t=w340, s=w341, f=w339) -> (s? t:f=w331:i16)
            n153 = Select(t=w330, s=w332, f=w331) -> (s? t:f=w329:i16)
            n154 = Select(t=w330, s=w333, f=w329) -> (s? t:f=w325:i16)
            n155 = Select(t=w325, s=w327, f=w324) -> (s? t:f=w326:i16)
            n156 = feedback-in #15(w326) -> ()
            n157 = feedback #16(w323) -> (w337:u64)
            n158 = Select(t=w323, s=w338, f=w337) -> (s? t:f=w312:u64)
            n159 = Increment(x=w312) -> (x+1=w334:u64)
            n160 = Select(t=w312, s=w327, f=w334) -> (s? t:f=w313:u64)
            n161 = Greater?(x="Number of scans (MCL)", y=w313) -> (0:w320:bool)
            n162 = Multiply(x="Scan freq.  increment (MCL)", y=w330) -> (x*y=w353:i16)
            n163 = Select(t=TRUE, s="Cont. Scan (MCL)", f=w320) -> (s? t:f=w319:bool)
            "Scanning MCL" <- w319
            n164 = Select(t=w313, s=w319, f=w323) -> (s? t:f=w335:u64)
            n165 = feedback-in #16(w335) -> ()
            n166 = Increment(x=w313) -> (x+1=→"Scan I (MCL)":u64)
            n167 = To Word Integer(number=w312) -> (16bit integer=w315:i16)
            n168 = Multiply(x=w315, y="Scan freq.  increment (MCL)") -> (x*y=w314:i16)
          }
        }
        n169 = Select(t=w290, s="1D or 2D Scan?", f=i16 0) -> (s? t:f=w291:i16)
        n170 = Select(t=w306, s="MCL Scan Axis", f=w291) -> (s? t:f=w307:i16)
        n171 = Select(t=w291, s="MCL Scan Axis", f=w306) -> (s? t:f=w305:i16)
        n172 = Add(x="AO2 (X)", y=w305) -> (x+y=w294:i16)
        n173 = Add(x="AO1 (Y)", y=w307) -> (x+y=w295:i16)
      }
      frame #3 {
        n174 = feedback-in #17(w376) -> ()
        n175 = feedback #17(w376) -> (w375:u32)
        n176 = Boolean To (0,1)(Boolean="+ phase (MCL)") -> (0, 1=w367:i16)
        n177 = Subtract(x=w376, y=w375) -> (x-y=w374:u32)
        n178 = Multiply(x=w367, y="Phase count adjustment (MCL)") -> (x*y=w363:i16)
        n179 = Subtract(x=w374, y=w373) -> (x-y=w355:u32)
        n180 = Subtract(x="MCL count", y=w355) -> (x-y=w365:u32)
        n181 = feedback #18(i16 0) -> (w364:i16)
        n182 = Subtract(x=w364, y=w363) -> (x-y=w362:i16)
        "MCL Relative Phase" <- w362
        n183 = feedback-in #18(w362) -> ()
        n184 = Number To Boolean Array(number=w355) -> (Boolean array=w356:bool[])
        n185 = Or Array Elements(Boolean array=w356) -> (logical OR=w354:bool)
        n186 = Boolean To (0,1)(Boolean=w354) -> (0, 1=w361:i16)
        n187 = Add(x=w365, y=w363) -> (x+y=w369:u32)
        n188 = To Unsigned Byte Integer(number=w361) -> (unsigned 8bit integer=w358:u8)
        n189 = feedback #19(u8 0) -> (w359:u8)
        n190 = Add(x=w358, y=w359) -> (x+y=w357:u8)
        "MCL Late Counter" <- w357
        n191 = feedback-in #19(w357) -> ()
      }
    }
  }
  n192 = while "APD 2 Counter" {
    tunnel: w2 -> [_]
    stop <- FALSE stop-if-true
    n193 = flat-sequence {
      frame #0 {
        n194 = xnode "FPGA I/O Method Node"("FPGA I/O In"=refnum<k21> "Connector0/DIO1" ("APD 2 DO"), "Timeout"=-1) -> ()  [unwired: 2 out]
      }
      frame #1 {
        n195 = local read "APD1 int gate"() -> (w381:bool)
        n196 = case shown="True" w381 {
          frame False {
          }
          frame True {
            n197 = local read "APD2 out state"() -> (w382:bool)
            n198 = case shown="True" w382 {
              frame False {
                n199 = local read "APD 2 Counts 0"() -> (w384:u32)
                n200 = Increment(x=w384) -> (x+1=→"APD 2 Counts 0":u32)
              }
              frame True {
                n201 = local read "APD 2 Counts 1"() -> (w386:u32)
                n202 = Increment(x=w386) -> (x+1=→"APD 2 Counts 1":u32)
              }
            }
          }
        }
      }
    }
  }
  n203 = while "Green fluorescent laser interlacing (Current to IA 532 nm AOM ME amp)." {
    shift-right: [w392] -> _
    shift-left: w2 -> [w395]
    shift-right: [w389] -> _
    shift-left: i16 0 -> [w387]
    stop <- FALSE stop-if-true
    n204 = flat-sequence {
      tunnel: w395 -> [w398]
      tunnel: [w399] -> w394
      tunnel: [w398] -> w393
      tunnel: [w397] -> w388
      tunnel: w387 -> [w397]
      tunnel: [w402] -> w391
      tunnel: w394 -> [w402]
      tunnel: [w401] -> w390
      tunnel: w393 -> [w401]
      tunnel: w388 -> [w400]
      tunnel: [w415] -> w392
      tunnel: [w431] -> w389
      tunnel: w391 -> [w444]
      tunnel: w390 -> [w441]
      frame #0 {
        n205 = call "Loop Timer10"("Count(Ticks)"=w398) -> ("Tick Count(Ticks)"=w399:u32)
      }
      frame #1 {
        n206 = xnode "FPGA I/O Node"("Chassis2/Mod1/AO0"=w400) -> ()  [unwired: 1 in, 1 out]
      }
      frame #2 {
        n207 = local read "RF synth bd controls green"() -> (w406:bool)
        n208 = Subtract(x="Green interlace OFF count 2", y="Green int current ON count adj") -> (x-y=w424:u32)
        n209 = feedback-in #20(w444) -> ()
        n210 = feedback #20(w444) -> (w443:u32)
        n211 = Add(x="Green int current ON count adj", y="Green interlace ON count 2") -> (x+y=w425:u32)
        n212 = Subtract(x=w444, y=w443) -> (x-y=w442:u32)
        n213 = Subtract(x=w442, y=w441) -> (x-y=w408:u32)
        n214 = Not(x=w406) -> (.not. x?=w404:bool)
        n215 = Number To Boolean Array(number=w408) -> (Boolean array=w409:bool[])
        n216 = Boolean To (0,1)(Boolean="+ phase (GI) 2") -> (0, 1=w421:i16)
        n217 = Or Array Elements(Boolean array=w409) -> (logical OR=w407:bool)
        "GI Late?" <- w407
        n218 = Boolean To (0,1)(Boolean=w407) -> (0, 1=w414:i16)
        n219 = Multiply(x=w421, y="Phase count adjustment (GI) 2") -> (x*y=w417:i16)
        n220 = To Unsigned Word Integer(number=w414) -> (unsigned 16bit integer=w410:u16)
        n221 = feedback #21(u16 0) -> (w412:u16)
        n222 = Add(x=w410, y=w412) -> (x+y=w411:u16)
        "GI Late Counter 2" <- w411
        n223 = feedback-in #21(w411) -> ()
        n224 = feedback #22(i16 0) -> (w418:i16)
        n225 = Subtract(x=w418, y=w417) -> (x-y=w416:i16)
        "GI Relative phase 2" <- w416
        n226 = feedback-in #22(w416) -> ()
        n227 = feedback #23(TRUE) -> (w436:bool)
        n228 = case shown="2" "Operating Mode 2" {
          tunnel: [TRUE FALSE w461] -> w426
          tunnel: w436 -> [_ _ w458]
          frame 0, Default {
          }
          frame 1 {
          }
          frame 2 {
            n229 = Not(x=w458) -> (.not. x?=w460:bool)
            n230 = Select(t=w460, s="Invert GI 2", f=w458) -> (s? t:f=w461:bool)
          }
        }
        n231 = And(x=w426, y="Green FB On/Off") -> (x .and. y?=w405:bool)
        "green FB running" <- w405
        n232 = And(x=w405, y=w404) -> (x .and. y?=w403:bool)
        n233 = case shown="True" w403 {
          tunnel: "Current Out" -> [w445 _]
          tunnel: [w445 w450] -> w430
          frame False {
          }
          frame True {
            n234 = local read "Green FB Sum"() -> (w446:i16)
            n235 = call "Slower PID.vi"("process variable"=w446, "reset?"="Green FB Reset", "setpoint"="Green FB Setpoint", "PID gains (x 2^8)"="Green FB Gains", "output range"=cluster{"output high":i16, "output low":i16} {"output high"=32767, "output low"=-32768} ("Green FB output range")) -> ("output"=w454:i16)  [unwired: 10 out]
            n236 = To Long Integer(number=w454) -> (32bit integer=w447:i32)
            n237 = Add(x=w447, y=32768) -> (x+y=w449:i32)
            n238 = To Unsigned Word Integer(number=w449) -> (unsigned 16bit integer=w450:u16)
          }
        }
        n239 = Not(x=w436) -> (.not. x?=w433:bool)
        n240 = Select(t=w425, s=w433, f=w424) -> (s? t:f=w438:u32)
        n241 = Subtract(x=w438, y=w408) -> (x-y=w419:u32)
        n242 = Add(x=w419, y=w417) -> (x+y=w415:u32)
        n243 = feedback-in #23(w433) -> ()
        n244 = Boolean To (0,1)(Boolean=w426) -> (0, 1=w432:i16)
        n245 = To Unsigned Word Integer(number=w432) -> (unsigned 16bit integer=w429:u16)
        n246 = Multiply(x=w429, y=w430) -> (x*y=w431:u16)
      }
    }
  }
  n247 = while "APD 1 Counter" {
    tunnel: w2 -> [_]
    stop <- FALSE stop-if-true
    n248 = flat-sequence {
      frame #0 {
        n249 = xnode "FPGA I/O Method Node"("FPGA I/O In"=refnum<k21> "Connector0/DIO0" ("APD 1 DO"), "Timeout"=-1) -> ()  [unwired: 2 out]
      }
      frame #1 {
        n250 = local read "APD1 int gate"() -> (w465:bool)
        n251 = case shown="True" w465 {
          frame False {
          }
          frame True {
            n252 = local read "APD1 out state"() -> (w466:bool)
            n253 = case shown="True" w466 {
              frame False {
                n254 = local read "APD 1 Counts 0"() -> (w468:u32)
                n255 = Increment(x=w468) -> (x+1=→"APD 1 Counts 0":u32)
              }
              frame True {
                n256 = local read "APD 1 Counts 1"() -> (w470:u32)
                n257 = Increment(x=w470) -> (x+1=→"APD 1 Counts 1":u32)
              }
            }
          }
        }
      }
    }
  }
  n258 = while "RF synth board interlacing timing loop" {
    tunnel: w2 -> [_]
    stop <- FALSE stop-if-true
    # "This loop is stalled until the RF FIFO get a value. With this method we gain additional delay time (because  we allow the rest of the main RF loop to procede while this loop waits to send the switch signals - a form of parallelism). This helps to simplify the main RF code. \n\nThe code also allow optimal interlacing while also controlling trap RF phase. \n\nNote: a lot of work has gone into optimizing these methods and it is unclear how they can be made any faster or better than this (many failed tries). Right now there is essentially ~4 ticks (~90 ns ns) of imperfection in the switching from trap 1 to trap 2. ~2 ticks of no RF (phase reset) then ~2 ticks of trap 2 with the wrong amplitude (T1 amplitude). The total ticks is 200, so not a big error.\n\nPhase can be precisely set for each trap. Phase reset and switching, has similar delays as fsk frequency switching. And phase reset and phase offset changes are also not simultaneous. So we can't perfectly line everything up.\n\nIf you start from amp zero though (as for trap 1), the on switch is perfect. Likewise the off is perfect for trap 2. \n\nThe green laser switching is also perfect because of its reduced duty cycle and delays in fsk switching between 80 and 0 MHz."
    n259 = xnode ("FIFO Read")("Timeout"=-1) -> ("Element"=w517:u16, "FIFO Out"=w513:refnum<k21>)  [unwired: 1 in, 1 out]
    n260 = Equal To 0?(x=w517) -> (x = 0?=w514:bool)
    n261 = Not(x=w514) -> (.not. x?=w471:bool)
    n262 = flat-sequence "BD 1 and 2 RF phase and amplitude switching" {
      tunnel: w471 -> [_]
      tunnel: w506 -> [w621]
      tunnel: w505 -> [w620]
      tunnel: w504 -> [w619]
      tunnel: w503 -> [w618]
      tunnel: w502 -> [w617]
      tunnel: w501 -> [w616]
      tunnel: w500 -> [w615]
      tunnel: w499 -> [w614]
      tunnel: w497 -> [w613]
      tunnel: w496 -> [w612]
      tunnel: w495 -> [w611]
      tunnel: w493 -> [w609]
      tunnel: w492 -> [w608]
      tunnel: w491 -> [w607]
      tunnel: w494 -> [w610]
      tunnel: w498 -> [w606]
      tunnel: w490 -> [w645]
      tunnel: w489 -> [w644]
      tunnel: w488 -> [w643]
      tunnel: w487 -> [w642]
      tunnel: w486 -> [w641]
      tunnel: w485 -> [w640]
      tunnel: w484 -> [w639]
      tunnel: w483 -> [w638]
      tunnel: w482 -> [w637]
      tunnel: w480 -> [w636]
      tunnel: w479 -> [w635]
      tunnel: w478 -> [w634]
      tunnel: w477 -> [w633]
      tunnel: w476 -> [w632]
      tunnel: w475 -> [w631]
      tunnel: w481 -> [w630]
      frame #0 {
        # "Delay to align amp/frequency switching depending on the method used.\n\nCan also give enough time to do the parallel amplitude calculations"
        n263 = call "Wait2"("Count(Ticks)"="Amp switch delay") -> ()  [unwired: 1 out]
      }
      frame #1 {
        w601 = TRUE ("Connector1/DIO30")
        # "make phase offset and phase reset active with buffer transfer"
        n264 = xnode "FPGA I/O Node"("Connector1/DIO29"=w601, "Connector1/DIO30"=w601) -> ()  [unwired: 2 in, 2 out]
      }
      frame #2 {
        w602 = FALSE ("Connector1/DIO15")
        # "write phase restart to buffer and reset udclk"
        n265 = xnode "FPGA I/O Node"("Connector1/DIO29"=w602, "Connector1/DIO30"=w602, "Connector1/DIO15"=FALSE ("Connector1/DIO14")) -> ()  [unwired: 3 in, 3 out]
      }
      frame #3 {
        w604 = TRUE ("Connector1/DIO15")
        # "make phase restart active"
        # "reset WR"
        n266 = xnode "FPGA I/O Node"("Connector1/DIO15"=w604, "Connector1/DIO29"=w604, "Connector1/DIO30"=w604) -> ()  [unwired: 3 in, 3 out]
      }
      frame #4 {
        w605 = FALSE ("Connector1/DIO30")
        # "Address"
        # "set amp byte 1, and reset udclk"
        n267 = xnode "FPGA I/O Node"("Connector1/DIO0"=w621, "Connector1/DIO1"=w620, "Connector1/DIO2"=w619, "Connector1/DIO3"=w618, "Connector1/DIO4"=w617, "Connector1/DIO5"=w616, "Connector1/DIO6"=w615, "Connector1/DIO7"=w614, "Connector1/DIO8"=TRUE, "Connector1/DIO9"=FALSE, "Connector1/DIO10"=FALSE, "Connector1/DIO11"=FALSE, "Connector1/DIO12"=FALSE, "Connector1/DIO13"=TRUE, "Connector1/DIO20"=w606, "Connector1/DIO21"=w613, "Connector1/DIO22"=w612, "Connector1/DIO23"=w611, "Connector1/DIO24"=w610, "Connector1/DIO25"=w609, "Connector1/DIO26"=w608, "Connector1/DIO27"=w607, "Connector1/DIO30"=w605, "Connector1/DIO29"=w605) -> ()  [unwired: 24 in, 24 out]
      }
      frame #5 {
        # "write amp byte 1 to buffer"
        n268 = xnode "FPGA I/O Node"("Connector1/DIO15"=FALSE ("Connector1/DIO14")) -> ()  [unwired: 1 in, 1 out]
      }
      frame #6 {
        # "reset WR"
        n269 = xnode "FPGA I/O Node"("Connector1/DIO15"=TRUE) -> ()  [unwired: 1 in, 1 out]
      }
      frame #7 {
        # "Address"
        # "set amp byte 2"
        n270 = xnode "FPGA I/O Node"("Connector1/DIO0"=w645, "Connector1/DIO1"=w644, "Connector1/DIO2"=w643, "Connector1/DIO3"=w642, "Connector1/DIO4"=w641, "Connector1/DIO5"=w640, "Connector1/DIO6"=w639, "Connector1/DIO7"=w638, "Connector1/DIO8"=TRUE, "Connector1/DIO9"=FALSE, "Connector1/DIO10"=FALSE, "Connector1/DIO11"=FALSE, "Connector1/DIO12"=TRUE, "Connector1/DIO13"=FALSE, "Connector1/DIO20"=w637, "Connector1/DIO21"=w630, "Connector1/DIO22"=w636, "Connector1/DIO23"=w635, "Connector1/DIO24"=w634, "Connector1/DIO25"=w633, "Connector1/DIO26"=w632, "Connector1/DIO27"=w631) -> ()  [unwired: 22 in, 22 out]
      }
      frame #8 {
        # "write amp byte 2"
        n271 = xnode "FPGA I/O Node"("Connector1/DIO15"=FALSE ("Connector1/DIO14")) -> ()  [unwired: 1 in, 1 out]
      }
      frame #9 {
        w653 = TRUE ("Connector1/DIO15")
        # "transfer amp bytes 1 and 2 and reset WR"
        n272 = xnode "FPGA I/O Node"("Connector1/DIO29"=w653, "Connector1/DIO30"=w653, "Connector1/DIO15"=TRUE ("Connector1/DIO14")) -> ()  [unwired: 3 in, 3 out]
      }
      frame #10 {
        w655 = FALSE ("Connector1/DIO14")
        # "reset udclk"
        n273 = xnode "FPGA I/O Node"("Connector1/DIO29"=w655, "Connector1/DIO30"=w655) -> ()  [unwired: 2 in, 2 out]
      }
    }
    n274 = flat-sequence "FSK BD 1 (trap X)" {
      tunnel: w471 -> [w519]
      tunnel: [w519] -> w474
      tunnel: w474 -> [w520]
      frame #0 {
        n275 = call "Wait"("Count(Ticks)"="BD 1 Delay (ticks)") -> ()  [unwired: 1 out]
      }
      frame #1 {
        # "switch frequency"
        n276 = xnode "FPGA I/O Node"("Connector1/DIO36"=w520) -> ()  [unwired: 1 in, 1 out]
      }
    }
    n277 = flat-sequence "FSK BD 2 (trap Y or green laser AOM)" {
      tunnel: w471 -> [w657]
      tunnel: [w657] -> w516
      tunnel: w516 -> [w658]
      frame #0 {
        n278 = call "Wait3"("Count(Ticks)"="BD 2 Delay (Ticks)") -> ()  [unwired: 1 out]
      }
      frame #1 {
        # "switch frequency"
        n279 = xnode "FPGA I/O Node"("Connector1/DIO37"=w658) -> ()  [unwired: 1 in, 1 out]
      }
    }
    n280 = xnode ("FIFO Read")("Timeout"=-1, "FIFO In"=w513) -> ("Element"=w508:u16, "FIFO Out"=w512:refnum<k21>)  [unwired: 1 out]
    n281 = xnode ("FIFO Read")("Timeout"=-1, "FIFO In"=w512) -> ("Element"=w507:u16)  [unwired: 2 out]
    n282 = node-c288() -> (w510:T7)  [unwired: 1 in]
    n283 = timed-loop "Convert amplitude words to bits" {
      timing: w510 -> [_]
      timing-out: [_] -> w509
      tunnel: w508 -> [w577]
      tunnel: w507 -> [w576]
      tunnel: [w553] -> w506
      tunnel: [w552] -> w505
      tunnel: [w551] -> w504
      tunnel: [w550] -> w503
      tunnel: [w549] -> w502
      tunnel: [w548] -> w501
      tunnel: [w547] -> w500
      tunnel: [w546] -> w499
      tunnel: [w545] -> w498
      tunnel: [w544] -> w497
      tunnel: [w543] -> w496
      tunnel: [w542] -> w495
      tunnel: [w541] -> w494
      tunnel: [w540] -> w493
      tunnel: [w539] -> w492
      tunnel: [w538] -> w491
      tunnel: [w537] -> w490
      tunnel: [w536] -> w489
      tunnel: [w535] -> w488
      tunnel: [w534] -> w487
      tunnel: [w533] -> w486
      tunnel: [w532] -> w485
      tunnel: [w531] -> w484
      tunnel: [w530] -> w483
      tunnel: [w529] -> w482
      tunnel: [w528] -> w481
      tunnel: [w527] -> w480
      tunnel: [w526] -> w479
      tunnel: [w525] -> w478
      tunnel: [w524] -> w477
      tunnel: [w523] -> w476
      tunnel: [w522] -> w475
      stop <- TRUE stop-if-true
      # "Board 1 Data"
      # "Board 2 Data"
      # "Board 1 Data"
      # "Board 2 Data"
      n284 = Split Number(x=w577) -> (hi(x)=w575:u8, lo(x)=w555:u8)
      n285 = Split Number(x=w576) -> (hi(x)=w574:u8, lo(x)=w554:u8)
      n286 = Number To Boolean Array(number=w575) -> (Boolean array=w595:bool[])
      n287 = Number To Boolean Array(number=w574) -> (Boolean array=w586:bool[])
      n288 = Index Array(array=w595, index=7) -> (element=w553:bool)
      n289 = Index Array(array=w595, index=6) -> (element=w552:bool)
      n290 = Index Array(array=w595, index=5) -> (element=w551:bool)
      n291 = Index Array(array=w595, index=4) -> (element=w550:bool)
      n292 = Index Array(array=w595, index=3) -> (element=w549:bool)
      n293 = Index Array(array=w595, index=2) -> (element=w548:bool)
      n294 = Index Array(array=w595, index=1) -> (element=w547:bool)
      n295 = Index Array(array=w595, index=0) -> (element=w546:bool)
      n296 = Index Array(array=w586, index=7) -> (element=w545:bool)
      n297 = Index Array(array=w586, index=6) -> (element=w544:bool)
      n298 = Index Array(array=w586, index=5) -> (element=w543:bool)
      n299 = Index Array(array=w586, index=4) -> (element=w542:bool)
      n300 = Index Array(array=w586, index=3) -> (element=w541:bool)
      n301 = Index Array(array=w586, index=2) -> (element=w540:bool)
      n302 = Index Array(array=w586, index=1) -> (element=w539:bool)
      n303 = Index Array(array=w586, index=0) -> (element=w538:bool)
      n304 = Number To Boolean Array(number=w555) -> (Boolean array=w573:bool[])
      n305 = Number To Boolean Array(number=w554) -> (Boolean array=w564:bool[])
      n306 = Index Array(array=w573, index=7) -> (element=w537:bool)
      n307 = Index Array(array=w573, index=6) -> (element=w536:bool)
      n308 = Index Array(array=w573, index=5) -> (element=w535:bool)
      n309 = Index Array(array=w573, index=4) -> (element=w534:bool)
      n310 = Index Array(array=w573, index=3) -> (element=w533:bool)
      n311 = Index Array(array=w573, index=2) -> (element=w532:bool)
      n312 = Index Array(array=w573, index=1) -> (element=w531:bool)
      n313 = Index Array(array=w573, index=0) -> (element=w530:bool)
      n314 = Index Array(array=w564, index=7) -> (element=w529:bool)
      n315 = Index Array(array=w564, index=6) -> (element=w528:bool)
      n316 = Index Array(array=w564, index=5) -> (element=w527:bool)
      n317 = Index Array(array=w564, index=4) -> (element=w526:bool)
      n318 = Index Array(array=w564, index=3) -> (element=w525:bool)
      n319 = Index Array(array=w564, index=2) -> (element=w524:bool)
      n320 = Index Array(array=w564, index=1) -> (element=w523:bool)
      n321 = Index Array(array=w564, index=0) -> (element=w522:bool)
    }
    n322 = node-c288(w509) -> ()
  }
  n323 = while "APD 1 Gating" {
    shift-right: [w662] -> _
    shift-left: w2 -> [w667]
    shift-right: [w661] -> _
    shift-left: w4 -> [w659]
    stop <- FALSE stop-if-true
    n324 = flat-sequence {
      tunnel: w667 -> [w670]
      tunnel: [w671] -> w665
      tunnel: [w670] -> w663
      tunnel: [w669] -> w660
      tunnel: w659 -> [w669]
      tunnel: [w674] -> w666
      tunnel: w665 -> [w674]
      tunnel: [w673] -> w664
      tunnel: w663 -> [w673]
      tunnel: w660 -> [w672]
      tunnel: [w694] -> w662
      tunnel: w666 -> [w708]
      tunnel: w664 -> [w705]
      tunnel: [w676] -> w661
      frame #0 {
        n325 = call "Loop Timer4"("Count(Ticks)"=w670) -> ("Tick Count(Ticks)"=w671:u32)
      }
      frame #1 {
        # "Signal maybe then sent through \na transistor before APD"
        n326 = xnode "FPGA I/O Node"("Connector1/DIO33"=w672) -> ()  [unwired: 1 in, 1 out]
        "APD1 int gate" <- w672
      }
      frame #2 {
        n327 = feedback #24(TRUE) -> (w700:bool)
        n328 = feedback-in #25(w708) -> ()
        n329 = feedback #25(w708) -> (w707:u32)
        n330 = Not(x=w700) -> (.not. x?=w697:bool)
        n331 = feedback-in #24(w697) -> ()
        n332 = Subtract(x=w708, y=w707) -> (x-y=w706:u32)
        n333 = Select(t="APD Gate ON Count", s=w697, f="APD Gate OFF Count") -> (s? t:f=w702:u16)
        n334 = Subtract(x=w706, y=w705) -> (x-y=w682:u32)
        n335 = Subtract(x=w702, y=w682) -> (x-y=w693:u32)
        n336 = Number To Boolean Array(number=w682) -> (Boolean array=w683:bool[])
        n337 = Or Array Elements(Boolean array=w683) -> (logical OR=w681:bool)
        n338 = Boolean To (0,1)(Boolean="+ phase (APD 1 Gate)") -> (0, 1=w691:i16)
        n339 = Boolean To (0,1)(Boolean=w681) -> (0, 1=w688:i16)
        n340 = Multiply(x=w691, y="Phase count adjustment (APD 1 Gate)") -> (x*y=w689:i16)
        n341 = To Unsigned Byte Integer(number=w688) -> (unsigned 8bit integer=w685:u8)
        n342 = Add(x=w693, y=w689) -> (x+y=w694:u32)
        n343 = feedback #26(i16 0) -> (w696:i16)
        n344 = Subtract(x=w696, y=w689) -> (x-y=w695:i16)
        "APD 1 Gate Relative Phase" <- w695
        n345 = feedback-in #26(w695) -> ()
        n346 = feedback #27(u8 0) -> (w686:u8)
        n347 = Add(x=w685, y=w686) -> (x+y=w684:u8)
        "APD 1 Gate Late Counter" <- w684
        n348 = feedback-in #27(w684) -> ()
        n349 = local read "Green long-scale interlacing"() -> (w675:bool)
        n350 = case shown="2" "APD Gate Operating Mode" {
          tunnel: [TRUE FALSE w730] -> w678
          tunnel: w700 -> [_ _ w730]
          frame 0, Default {
          }
          frame 1 {
          }
          frame 2 {
          }
        }
        n351 = Not(x=w678) -> (.not. x?=w679:bool)
        n352 = Select(t=w679, s="Invert APD Gate", f=w678) -> (s? t:f=w677:bool)
        n353 = case shown="True" w675 {
          tunnel: w677 -> [w709 w717]
          tunnel: [w709 w718] -> w676
          frame False {
          }
          frame True {
            n354 = local read "Number of ON cycles"() -> (w711:i16)
            n355 = local read "Number of OFF cycles"() -> (w713:i16)
            n356 = feedback #28(i16 1) -> (w724:i16)
            n357 = Increment(x=w724) -> (x+1=w723:i16)
            n358 = feedback #29(w711) -> (w710:i16)
            n359 = Greater?(x=w710, y=w724) -> (0:w719:bool)
            n360 = Select(t=w723, s=w719, f=i16 1) -> (s? t:f=w721:i16)
            n361 = feedback-in #28(w721) -> ()
            n362 = feedback #30(TRUE) -> (w716:bool)
            n363 = Not(x=w716) -> (.not. x?=w715:bool)
            n364 = Select(t=w716, s=w719, f=w715) -> (s? t:f=w714:bool)
            n365 = feedback-in #30(w714) -> ()
            n366 = Select(t=w711, s=w714, f=w713) -> (s? t:f=w712:i16)
            n367 = feedback-in #29(w712) -> ()
            n368 = case shown="True" w714 {
              tunnel: [FALSE w727] -> w718
              tunnel: w717 -> [_ w727]
              frame False {
              }
              frame True {
              }
            }
          }
        }
      }
    }
  }
  n369 = while "Trap RF control, main calculations (raster scanning, intensity and position feedback, phase control etc) with primary timing trigger" {
    shift-right: [w745] -> _
    shift-left: w2 -> [w744]
    shift-right: [w743] -> _
    shift-left: FALSE ("Swap F1 and F2") -> [w742]
    shift-right: [w738] -> _
    shift-left: u16 0 ("BD 1 Amplitude 3") -> [w735]
    shift-right: [w737] -> _
    shift-left: u16 0 ("BD 2 Amplitude 3") -> [w733]
    shift-right: [w732] -> _
    shift-left: u64 0 -> [w731]
    stop <- FALSE stop-if-true
    n370 = flat-sequence {
      tunnel: w742 -> [w751]
      tunnel: w744 -> [w748]
      tunnel: [w751] -> w741
      tunnel: [w747] -> w740
      tunnel: [w748] -> w739
      tunnel: [w750] -> w736
      tunnel: w735 -> [w750]
      tunnel: [w749] -> w734
      tunnel: w733 -> [w749]
      tunnel: [w762] -> w745
      tunnel: [w761] -> w743
      tunnel: w741 -> [w760]
      tunnel: w740 -> [w759]
      tunnel: w739 -> [w758]
      tunnel: [w757] -> w738
      tunnel: [w756] -> w737
      tunnel: w736 -> [w755]
      tunnel: w734 -> [w754]
      tunnel: [w753] -> w732
      tunnel: w731 -> [w752]
      frame #0 {
        n371 = call "Loop Timer2"("Count(Ticks)"=w748) -> ("Tick Count(Ticks)"=w747:u32)
      }
      frame #1 {
        n372 = flat-sequence {
          tunnel: w760 -> [w770]
          tunnel: w755 -> [w764]
          tunnel: w754 -> [w763]
          tunnel: [w830] -> w762
          tunnel: [w842] -> w761
          tunnel: w759 -> [w836]
          tunnel: w758 -> [w833]
          tunnel: [w781] -> w757
          tunnel: [w780] -> w756
          tunnel: [w772] -> w753
          tunnel: w752 -> [w771]
          frame #0 {
            w765 = -1 ("Timeout")
            # "Operation when you need a long delay for either X or Y to synchonize AOD light out phase (> ~100 ticks)\nor want shorter trap ON timing. Puts some of the delay timing in parallel with the later computations."
            # "Trigger the external loop by sending the boolean FSK value through a FIFO.\nTiming is precise."
            n373 = Boolean To (0,1)(Boolean=w770) -> (0, 1=w769:i16)
            n374 = To Unsigned Word Integer(number=w769) -> (unsigned 16bit integer=w768:u16)
            n375 = xnode ("FIFO Method Node")("Element"=w768, "Timeout"=w765) -> ("FIFO Out"=w767:refnum<k21>)  [unwired: 1 in, 1 out]
            n376 = xnode ("FIFO Method Node")("Element"=w764, "Timeout"=w765, "FIFO In"=w767) -> ("FIFO Out"=w766:refnum<k21>)  [unwired: 1 out]
            n377 = xnode ("FIFO Method Node")("Element"=w763, "Timeout"=w765, "FIFO In"=w766) -> ()  [unwired: 2 out]
          }
          frame #1 {
            # "Just counts, wraps around, 8 bit"
            # "Which trap cycle"
            # "Only save the 3rd set's amp in the loop"
            # "If this is NOT set 3 AND NOT (RF synth controls green AND green FB running)\nthen use this sets amp value (otherwise keep the green feedback value)"
            # "Just flips back and forth."
            # "If interlacing is off, this is which cycle to use."
            # "Keep track of trap cycles (trap 1, 2, 3...)"
            # "This is the prior cycle's on time"
            # "increment timing\nindex, reset to 0 if \nend of matrix"
            # "Reset to begginning (1) when number of cycles reached."
            # "timing index"
            # "build byte stacks for writing data\n(must correspond to addresses array constant)"
            # "Timing housekeeping"
            # "Adjust phase if late\n(maintains constant phase relationship between cycles)"
            n378 = feedback #31(u8 0 ("t")) -> (w839:u8)
            n379 = Increment(x=w839) -> (x+1=w878:u8)
            n380 = Increment(x="Number Interlace Cycles") -> (x+1=w873:u8)
            n381 = Equal?(x=w878, y=w873) -> (x = y?=w880:bool)
            n382 = Select(t=u8 1, s=w880, f=w878) -> (s? t:f=w838:u8)
            n383 = feedback-in #31(w838) -> ()
            n384 = Increment(x=w838) -> (x+1=w875:u8)
            n385 = Equal?(x=w875, y=w873) -> (x = y?=w876:bool)
            n386 = Select "This cycle"(t=u8 1, s=w876, f=w875) -> (s? t:f=w872:u8)
            n387 = Select(t=w872, s="Interlace ON/OFF", f="Interlace Off Parameters") -> (s? t:f=w791:u8)
            n388 = feedback-in #32(w836) -> ()
            n389 = feedback #32(w836) -> (w835:u32)
            n390 = Select(t=w838, s="Interlace ON/OFF", f="Interlace Off Parameters") -> (s? t:f=w871:u8)
            n391 = Subtract(x=w836, y=w835) -> (x-y=w834:u32)
            n392 = Subtract "The error"(x=w834, y=w833) -> (x-y=w817:u32)
            n393 = case shown="1, Default" w871 {
              tunnel: ["DIO count 1 (ticks)" "DIO count 2 (ticks)" "DIO count 3 (ticks)"] -> w832
              frame 1, Default {
              }
              frame 2 {
              }
              frame 3 {
              }
            }
            n394 = Number To Boolean Array(number=w817) -> (Boolean array=w818:bool[])
            n395 = Or Array Elements(Boolean array=w818) -> (logical OR=w816:bool)
            n396 = Boolean To (0,1)(Boolean=w816) -> (0, 1=w823:i16)
            n397 = To Unsigned Byte Integer(number=w823) -> (unsigned 8bit integer=w820:u8)
            n398 = feedback #33(u8 0) -> (w821:u8)
            n399 = Add(x=w820, y=w821) -> (x+y=w819:u8)
            "DIO Late Counter" <- w819
            n400 = feedback-in #33(w819) -> ()
            n401 = Subtract(x=w832, y=w817) -> (x-y=w831:u32)
            n402 = disable-structure shown="Disabled" {
              disable-tunnel: [w884 _] -> w815
              disable-tunnel: w791 -> [w881 _]
              frame Disabled {
                n403 = feedback #34(i64 0 ("y")) -> (w883:i64)
                n404 = case "Synchronize trap oscillations - always begin/end with trap 1" shown="1, Default" w881 {
                  tunnel: [w885 w886 w887] -> w884
                  tunnel: w883 -> [w885 w886 _]
                  frame 2 {
                  }
                  frame 3 {
                  }
                  frame 1, Default {
                    n405 = Or(x="Osc traps", y="Initiate trap osc") -> (x .or. y?=w889:bool)
                    n406 = case "Trap sine oscillation (or whatever pattern is stored in memory)" shown="True" w889 {
                      tunnel: [i64 0 ("y") w893] -> w887
                      tunnel: "Initiate trap osc" -> [_ w896]
                      frame False {
                      }
                      frame True {
                        w900 = u16 0
                        w898 = -1
                        n407 = local write "Initiate trap osc"(FALSE ("Initiate trap osc")) -> ()
                        n408 = feedback #35(w900) -> (w902:u16)
                        n409 = Select(t=w900, s=w896, f=w902) -> (s? t:f=w901:u16)
                        n410 = Greater Or Equal?(x=w901, y="Trap osc period (pts)") -> (x >= y?=w907:bool)
                        n411 = Or(x=w896, y=w907) -> (x .or. y?=w908:bool)
                        n412 = Select(t=u16 0, s=w908, f=w901) -> (s? t:f=w892:u16)
                        n413 = feedback #36(w898) -> (w899:i32)
                        n414 = Select(t=w898, s=w896, f=w899) -> (s? t:f=w897:i32)
                        n415 = Increment(x=w897) -> (x+1=w904:i32)
                        n416 = Equal?(x=w892, y=u16 0) -> (x = y?=w905:bool)
                        n417 = Increment(x=w892) -> (x+1=w912:u16)
                        n418 = feedback-in #35(w912) -> ()
                        n419 = Select(t=w904, s=w905, f=w897) -> (s? t:f=w903:i32)
                        n420 = feedback-in #36(w903) -> ()
                        n421 = case shown="False" "Osc trap cont." {
                          tunnel: w903 -> [w916 _]
                          frame False {
                            n422 = Greater Or Equal?(x=w916, y="N trap osc periods") -> (x >= y?=w914:bool)
                            n423 = Not(x=w914) -> (.not. x?=w913:bool)
                            n424 = local write "Osc traps"(w913) -> ()
                          }
                          frame True {
                          }
                        }
                        n425 = xnode ("Memory Read")("Address"=w892, "Memory In"=refnum<k21> "Trap osc memory") -> ("Data"=w893:i64)  [unwired: 1 out]
                      }
                    }
                  }
                }
                n426 = feedback-in #34(w884) -> ()
              }
              frame Enabled {
              }
            }
            n427 = local read "green FB running"() -> (w804:bool)
            n428 = And(x=w804, y="RF synth bd controls green") -> (x .and. y?=w803:bool)
            n429 = case shown="1, Default" w791 {
              tunnel: [w1043 w1279 "BD 1 Frequency 3"] -> w868
              tunnel: [w1084 w1278 w1300] -> w807
              tunnel: ["BD 2 Amplitude 1" "BD 2 Amplitude 2" w1299] -> w799
              tunnel: [w1040 w1275 "BD 1 Amplitude 3"] -> w781
              tunnel: "FB Gains" -> [w1061 w1285 _]
              tunnel: "FB output range" -> [w1062 w1284 _]
              tunnel: w815 -> [w1059 w1282 _]
              tunnel: "BD 2 Frequency 1" -> [w1056 _ _]
              tunnel: "BD 2 Frequency 2" -> [_ w1278 _]
              tunnel: "BD 2 Frequency 3" -> [_ _ w1300]
              tunnel: w803 -> [_ _ w1298]
              tunnel: [w1043 w1276 w1297] -> w772
              tunnel: w771 -> [w1042 w1276 w1297]
              frame 1, Default {
                w1075 = fxp<+/-,24,9> 0.0 ("AI1 X Set 2")
                w1069 = u16 0
                w1082 = u64 0 ("f")
                # "Changed by Ronen - correction \nby PID is now implemented not on \nthe Base BD1 frequency but on the last\nfrequency sent."
                # "Added by Ronen -\nUpper and Lower \nLimits for the FB \ngenerated frequency\nto avoid losing bead \nwhen tether breaks"
                # "Explanation of raster scanning:\n1. Cycles: increment counter by 1 every time interlace cycle returns to trap 1. As long as \n  Cycle per Step is larger than counter, keep incrementing counter and do not change step counter.\n  Once counter is equal to Cycles per step, zero counter and increment step counter.\n2. Steps: Increments up every time cycles counter equals cycles per step. Performs the following:\n- To determine DIRECTION of frequency change:  If ScanstepX2 is EQUAL to step counter (full for-back scan finished)\n   frequency increment is set to zero, AND step counter is set to zero. \n   Otherwise: if no change to step counter (because cycleperstep>cycle counter), then no change to frequency\n   increment. \n   If step counter has changed (cycleperstep=cycle counter), then need to figure out direction of frequency change:\n   if step counter is EQUAL to Scansteps: No change to frequency increment\n   Otherwise: If scan steps > step counter - 1 (forward scan NOT completed): increment frequency by 1\n                       If scan steps equal or smaller than step counter -1 (forward scan completed): increment frequency by -1\n\n3. Scans: Increment scan counter every time step counter equals 2Xscan steps (full for-back scan completed)\n    if number of scans > scan counter: Send TRUE to scanning, continue scan\n    if number of scans = scan counter: Send FALSE to Scanning, Scan finished.\n\n  The wire with the asterik can be used as the index for getting the mirror positions in the offset scan."
                # "This signal integration happens no matter what\nso that correct setpoints can be chosen before \nturning on the FB."
                # "Trap 1"
                n430 = local read "AI1 X Set 2"() -> (w1054:fxp<+/-,16,1>)
                n431 = local read "AI1 X Set 1"() -> (w1072:fxp<+/-,16,1>)
                n432 = local read "Scanning"() -> (w1085:bool)
                n433 = Multiply(x=w1054, y="B factor") -> (x*y=w1052:fxp<+/-,48,17>)
                n434 = Or(x=w1085, y="Start scan") -> (x .or. y?=w1037:bool)
                n435 = case shown="True" "Diff FB Measurement?" {
                  tunnel: w1052 -> [w1175 w1184]
                  tunnel: w1072 -> [w1174 w1185]
                  tunnel: [w1172 w1176] -> w1073
                  frame False {
                    n436 = Select(t=w1174, s="Trap Pos FB Monitor T1 or T2", f=w1175) -> (s? t:f=w1172:fxp<+/-,48,17>)
                  }
                  frame True {
                    n437 = Subtract(x=w1185, y=w1184) -> (x-y=w1177:fxp<+/-,48,17>)
                    n438 = Not(x="Negate Diff?") -> (.not. x?=w1183:bool)
                    n439 = Boolean To (0,1)(Boolean="Negate Diff?") -> (0, 1=w1181:i16)
                    n440 = Boolean To (0,1)(Boolean=w1183) -> (0, 1=w1182:i16)
                    n441 = Negate(x=w1181) -> (-x=w1180:i16)
                    n442 = Add(x=w1180, y=w1182) -> (x+y=w1178:i16)
                    n443 = Multiply(x=w1178, y=w1177) -> (x*y=w1176:fxp<+/-,63,32>)
                  }
                }
                n444 = feedback #37(w1069) -> (w1068:u16)
                n445 = Increment(x=w1068) -> (x+1=w1070:u16)
                n446 = Greater Or Equal?(x=w1070, y="Trap Pos FB Int Count") -> (x >= y?=w1041:bool)
                n447 = Select(t=w1069, s=w1041, f=w1070) -> (s? t:f=w1071:u16)
                n448 = feedback-in #37(w1071) -> ()
                n449 = feedback #38(w1075) -> (w1074:fxp<+/-,24,9>)
                n450 = Add(x=w1073, y=w1074) -> (x+y=w1067:fxp<+/-,24,9>)
                n451 = Select(t=w1075, s=w1041, f=w1067) -> (s? t:f=w1078:fxp<+/-,24,9>)
                n452 = feedback-in #38(w1078) -> ()
                n453 = case "Trap 1 X intensity feedback" shown="True" "FB On/Off Set 1" {
                  tunnel: "BD 1 Amplitude 1" -> [w1267 _]
                  tunnel: [w1267 w1271] -> w1040
                  tunnel: w1062 -> [_ w1268]
                  tunnel: w1061 -> [_ w1269]
                  frame False {
                  }
                  frame True {
                    n454 = local read "AI2 Y Sum Set 1"() -> (w1272:i16)
                    n455 = call "Slower PID.vi"("process variable"=w1272, "reset?"="FB Reset Set 1", "setpoint"="FB Setpoint Set 1", "PID gains (x 2^8)"=w1269, "output range"=w1268) -> ("output"=w1273:i16)  [unwired: 10 out]
                    n456 = To Unsigned Word Integer(number=w1273) -> (unsigned 16bit integer=w1271:u16)
                  }
                }
                "BD1 amplitude 1 out" <- w1040
                n457 = Divide(x=w1067, y="Trap Pos FB Int Count") -> (x/y=w1038:fxp<+/-,16,1>)
                n458 = case "For raster scanning" shown="True" w1037 {
                  tunnel: [u64 0 w1115] -> w1039
                  tunnel: [FALSE w1103] -> w1032
                  tunnel: [i16 0 w1102] -> w1033
                  tunnel: w1038 -> [_ w1101]
                  tunnel: "Start scan" -> [_ w1095]
                  frame False {
                    n459 = local write "Scanning"(FALSE ("scanning")) -> ()
                  }
                  frame True {
                    w1109 = u64 0
                    # "Changed by RG, to introduce force\ndependent stopping of the raster scan \nand manual stopping"
                    # "count number of cycles"
                    n460 = feedback #39(w1109) -> (w1112:u64)
                    n461 = Select(t=w1109, s=w1095, f=w1112) -> (s? t:f=w1114:u64)
                    n462 = Increment(x=w1114) -> (x+1=w1107:u64)
                    n463 = Equal?(x=i16 1, y=w1107) -> (x = y?=w1105:bool)
                    n464 = And(x="Abort scan", y=w1105) -> (x .and. y?=w1103:bool)
                    n465 = Greater?(x="Cycles per step", y=w1107) -> (0:w1110:bool)
                    n466 = Select(t=w1107, s=w1110, f=w1109) -> (s? t:f=w1111:u64)
                    n467 = feedback-in #39(w1111) -> ()
                    n468 = Greater?(x=w1101, y="Raster setpoint") -> (0:w1098:bool)
                    n469 = And(x=w1098, y="Raster to target force") -> (x .and. y?=w1096:bool)
                    n470 = case shown="False" w1103 {
                      tunnel: [w1122 i16 0] -> w1115
                      tunnel: w1095 -> [w1147 _]
                      tunnel: w1110 -> [w1140 _]
                      tunnel: w1109 -> [w1130 _]
                      tunnel: [w1124 FALSE] -> w1104
                      tunnel: [w1120 w1158] -> w1102
                      tunnel: [w1123 w1159] -> w1099
                      frame False {
                        w1131 = i64 0
                        # "scan incr."
                        # "freq. incr. mult."
                        # "count steps"
                        n471 = feedback #40(w1130) -> (w1155:u64)
                        n472 = Select(t=w1130, s=w1147, f=w1155) -> (s? t:f=w1123:u64)
                        n473 = Increment(x=w1123) -> (x+1=w1154:u64)
                        n474 = Add(x="Scan steps", y="Scan steps") -> (x+y=w1153:u64)
                        n475 = Select(t=w1123, s=w1140, f=w1154) -> (s? t:f=w1135:u64)
                        n476 = Greater?(x=w1153, y=w1135) -> (0:w1134:bool)
                        n477 = Select(t=w1135, s=w1134, f=w1130) -> (s? t:f=w1151:u64)
                        n478 = feedback-in #40(w1151) -> ()
                        n479 = Equal?(x="Scan steps", y=w1135) -> (x = y?=w1139:bool)
                        n480 = Greater?(x="Scan steps", y=w1123) -> (0:w1150:bool)
                        n481 = feedback #41(w1131) -> (w1152:i64)
                        n482 = Select(t=w1131, s=w1147, f=w1152) -> (s? t:f=w1137:i64)
                        n483 = Increment(x=w1137) -> (x+1=w1149:i64)
                        n484 = Decrement(x=w1137) -> (x-1=w1148:i64)
                        n485 = Select(t=w1149, s=w1150, f=w1148) -> (s? t:f=w1138:i64)
                        n486 = Select(t=w1137, s=w1139, f=w1138) -> (s? t:f=w1136:i64)
                        n487 = Select(t=w1137, s=w1140, f=w1136) -> (s? t:f=w1132:i64)
                        n488 = Select(t=w1132, s=w1134, f=w1131) -> (s? t:f=w1133:i64)
                        n489 = feedback-in #41(w1133) -> ()
                        n490 = feedback #42(w1130) -> (w1146:u64)
                        n491 = Select(t=w1130, s=w1147, f=w1146) -> (s? t:f=w1142:u64)
                        n492 = Increment(x=w1142) -> (x+1=w1143:u64)
                        n493 = Select(t=w1142, s=w1134, f=w1143) -> (s? t:f=w1141:u64)
                        n494 = Greater?(x="Number of scans", y=w1141) -> (0:w1127:bool)
                        n495 = Multiply(x="Scan freq.  increment", y=w1137) -> (x*y=w1122:i64)
                        n496 = Select(t=TRUE, s="Cont. Scan", f=w1127) -> (s? t:f=w1124:bool)
                        n497 = Select(t=w1141, s=w1124, f=w1130) -> (s? t:f=w1144:u64)
                        n498 = feedback-in #42(w1144) -> ()
                        n499 = local read "BD 1 Frequency 1"() -> (w1121:u64)
                        n500 = Increment(x=w1141) -> (x+1=→"Scan I":u64)
                        n501 = Add(x=w1122, y=w1121) -> (x+y=w1120:u64)
                        "Actual Scan freq" <- w1120
                      }
                      frame True {
                        n502 = local read "Actual Scan freq"() -> (w1158:u64)
                        n503 = local read "Scan steps"() -> (w1159:u64)
                      }
                    }
                    "Scanning" <- w1104
                    n504 = case shown="True" w1096 {
                      tunnel: w1099 -> [_ w1119]
                      frame False {
                      }
                      frame True {
                        n505 = Add(x=w1119, y=i16 2) -> (x+y=w1117:u64)
                        n506 = local write "Raster to target force"(FALSE) -> ()
                        n507 = local write "Scan steps"(w1117) -> ()
                      }
                    }
                  }
                }
                n508 = feedback #43(fxp<+/-,24,9> 0.0 ("AI1 X Set 2")) -> (w1079:fxp<+/-,24,9>)
                n509 = Select(t=w1067, s=w1041, f=w1079) -> (s? t:f=w1080:fxp<+/-,24,9>)
                "Trap Pos FB Int Signal" <- w1080
                n510 = feedback-in #43(w1080) -> ()
                n511 = feedback #44(fxp<+/-,16,1> 0.0 ("Trap Pos FB Int-Norm Signal")) -> (w1064:fxp<+/-,16,1>)
                n512 = Select(t=w1038, s=w1041, f=w1064) -> (s? t:f=w1063:fxp<+/-,16,1>)
                "Trap Pos FB Int-Norm Signal" <- w1063
                n513 = feedback-in #44(w1063) -> ()
                n514 = case "For position feedback" shown="True" "Force feedback" {
                  tunnel: [i64 0 w1191] -> w1048
                  tunnel: w1038 -> [_ w1188]
                  tunnel: w1041 -> [_ w1187]
                  frame False {
                  }
                  frame True {
                    n515 = feedback #45(i64 0) -> (w1190:i64)
                    n516 = case shown="True" w1187 {
                      tunnel: [w1192 w1196] -> w1191
                      tunnel: w1190 -> [w1192 _]
                      tunnel: w1188 -> [_ w1195]
                      frame False {
                      }
                      frame True {
                        n517 = xnode ("PID")("process variable"=w1195, "reset?"="Trap Pos. FB Reset", "setpoint"="Trap Pos. FB SP", "PID gains"="Trap Pos. FB Gains", "output range"="Trap pos. FB Range") -> ("output"=w1205:fxp<+/-,16,1>)
                        n518 = Negate(x=w1205) -> (-x=w1204:fxp<+/-,17,2>)
                        n519 = Select(t=w1204, s="Trap Pos FB Negate Action", f=w1205) -> (s? t:f=w1201:fxp<+/-,17,2>)
                        n520 = Scale By Power Of 2(n=u32 15, x=u32 1) -> (x*2^n=w1198:u32)
                        n521 = Multiply(x=w1201, y=w1198) -> (x*y=w1197:fxp<+/-,17,17>)
                        n522 = To Quad Integer(1:w1197) -> (0:w1209:i64)
                        "Trap Pos FB Action" <- w1209
                        n523 = Multiply(x=w1209, y="Trap Pos. FB Mult Factor") -> (x*y=w1207:i64)
                        n524 = Add(x=w1207, y="Trap Pos. FB Offset Factor") -> (x+y=w1196:i64)
                        n525 = disable-structure shown="Disabled" {
                          disable-tunnel: w1196 -> [w1216 _]
                          frame Disabled {
                            w1220 = u32 0
                            n526 = feedback #46() -> (w1217:i64)  [unwired: 1 in]
                            n527 = Add(x=w1216, y=w1217) -> (x+y=w1214:i64)
                            n528 = feedback #47(w1220) -> (w1222:u32)
                            n529 = Increment(x=w1222) -> (x+1=w1211:u32)
                            n530 = Greater Or Equal?(x=w1211, y="FB Trig Integrate") -> (x >= y?=w1212:bool)
                            n531 = Select(t=i64 0, s=w1212, f=w1214) -> (s? t:f=w1218:i64)
                            n532 = feedback-in #46(w1218) -> ()
                            n533 = Select(t=w1220, s=w1212, f=w1211) -> (s? t:f=w1221:u32)
                            n534 = feedback-in #47(w1221) -> ()
                            n535 = And(x=w1212, y="FPGA Trap Trig") -> (x .and. y?=w1219:bool)
                            n536 = case "Trap FB trigger excitation laser ON" shown="True" w1219 {
                              tunnel: w1214 -> [_ w1226]
                              tunnel: w1211 -> [_ w1224]
                              frame False {
                              }
                              frame True {
                                n537 = Not(x="TTrig Negate Pos") -> (.not. x?=w1233:bool)
                                n538 = Boolean To (0,1)(Boolean="TTrig Negate Pos") -> (0, 1=w1231:i16)
                                n539 = Boolean To (0,1)(Boolean=w1233) -> (0, 1=w1232:i16)
                                n540 = Negate(x=w1231) -> (-x=w1230:i16)
                                n541 = Add(x=w1230, y=w1232) -> (x+y=w1229:i16)
                                n542 = Multiply(x=w1229, y=w1226) -> (x*y=w1228:i64)
                                "TTrig Sig" <- w1228
                                n543 = Multiply(x="FPGA TTrig Thresh", y=w1224) -> (x*y=w1225:i64)
                                "TTrig Fin Thresh" <- w1225
                                n544 = Greater Or Equal?(x=w1228, y=w1225) -> (x >= y?=w1227:bool)
                                n545 = case shown="True" w1227 {
                                frame False {
                                }
                                frame True {
                                w1236 = TRUE ("Green FB On/Off")
                                w1238 = u8 2 ("Operating Mode")
                                n546 = local write "Operating Mode"(w1238) -> ()
                                n547 = local write item#-1(w1238) -> ()
                                n548 = local write item#-1(w1236) -> ()
                                n549 = local write "FPGA Trap Trig"(FALSE ("FPGA Trap Trig")) -> ()
                                "TTrig?" <- w1236
                                }
                                }
                              }
                            }
                          }
                          frame Enabled {
                          }
                        }
                      }
                    }
                    n550 = feedback-in #45(w1191) -> ()
                  }
                }
                n551 = And(x="Force feedback", y="Dynamic Force FB (Ronen)") -> (x .and. y?=w1049:bool)
                n552 = case shown="True" w1049 {
                  tunnel: w1048 -> [w1163 w1167]
                  tunnel: [w1162 w1166] -> w1034
                  tunnel: w1042 -> [_ w1165]
                  tunnel: w1041 -> [_ w1164]
                  frame False {
                    # "(BD1 Frequency 1)"
                    n553 = Add(x="BD 1 Frequency 1", y=w1163) -> (x+y=w1162:u64)
                  }
                  frame True {
                    n554 = case shown="True" w1164 {
                      tunnel: w1167 -> [_ w1171]
                      tunnel: [w1168 w1170] -> w1166
                      tunnel: w1165 -> [w1168 w1169]
                      frame False {
                      }
                      frame True {
                        n555 = Add(x=w1169, y=w1171) -> (x+y=w1170:u64)
                      }
                    }
                  }
                }
                n556 = case shown="True" w1032 {
                  tunnel: [w1088 w1090] -> w1035
                  tunnel: w1034 -> [w1088 _]
                  tunnel: w1033 -> [_ w1090]
                  frame False {
                  }
                  frame True {
                    n557 = local write "BD 1 Frequency 1"(w1090) -> ()
                    n558 = local write "Abort scan"(FALSE) -> ()
                  }
                }
                n559 = Select(t=w1059, s="Trap 1 osc enable", f=i64 0) -> (s? t:f=w1057:i64)
                n560 = Select(t=w1082, s="Scan BD", f=w1039) -> (s? t:f=w1081:u64)
                n561 = Select(t=w1039, s="Scan BD", f=w1082) -> (s? t:f=w1047:u64)
                n562 = Add(x=w1081, y=w1056) -> (x+y=w1084:u64)
                n563 = Compound Arithmetic op=ADD(w1057, w1035, w1047) -> (w1046:u64)
                n564 = In Range and Coerce(upper limit="FB Max Frequency", x=w1046, lower limit="FB Min frequency") -> (coerced(x)=w1043:u64)  [unwired: 1 out]
                "BD1 Frequency Out 1" <- w1043
              }
              frame 2 {
                # "Trap 2"
                n565 = case "Trap 2 X intensity feedback" shown="True" "FB On/Off Set 2" {
                  tunnel: [w1289 w1292] -> w1275
                  tunnel: "BD 1 Amplitude 2" -> [w1289 _]
                  tunnel: w1285 -> [_ w1291]
                  tunnel: w1284 -> [_ w1290]
                  frame False {
                  }
                  frame True {
                    n566 = local read "AI2 Y Sum Set 2"() -> (w1295:i16)
                    n567 = call "Slower PID.vi"("process variable"=w1295, "reset?"="FB Reset Set 2", "setpoint"="FB Setpoint Set 2", "PID gains (x 2^8)"=w1291, "output range"=w1290) -> ("output"=w1293:i16)  [unwired: 10 out]
                    n568 = To Unsigned Word Integer(number=w1293) -> (unsigned 16bit integer=w1292:u16)
                  }
                }
                "BD1 amplitude 2 out" <- w1275
                n569 = Select(t=w1282, s="Trap 2 osc enable", f=i64 0) -> (s? t:f=w1281:i64)
                n570 = Add(x="BD 1 Frequency 2", y=w1281) -> (x+y=w1279:u64)
                "BD1 Frequency Out 2" <- w1279
              }
              frame 3 {
                # "Fluorescence period"
                n571 = disable-structure shown="Disabled" {
                  disable-tunnel: [w1308 _] -> w1299
                  disable-tunnel: w1298 -> [w1307 _]
                  frame Disabled {
                    # "Remember if FB was previously on/off"
                    n572 = feedback #48(FALSE) -> (w1303:bool)
                    n573 = case shown="True" w1307 {
                      tunnel: [w1310 w1326] -> w1308
                      tunnel: "BD 2 Amplitude 3" -> [w1310 _]
                      tunnel: [FALSE TRUE] -> w1304
                      tunnel: w1303 -> [_ w1312]
                      frame False {
                      }
                      frame True {
                        # "Makes it so first time FB run when turned on, the PID sees the detector intensity from the last time FB was running, rather than something near zero. Especially assuming the setpoint is not changing, this will make the FB more stable when resuming, and not overshoot the turnon intensity."
                        # "FB output range: 0 should be low, full scale is 12 bits.\nBut be careful not to go over, then higher bits just get ignored by RF board, so output will actually jump down and be unstable. Keep it under 4000 to be safe."
                        n574 = local read "Green FB Sum"() -> (w1311:i16)
                        n575 = feedback-in #49(w1311) -> ()
                        n576 = feedback #49(i16 0 ("Green FB Sum")) -> (w1314:i16)
                        n577 = Select(t=w1311, s=w1312, f=w1314) -> (s? t:f=w1313:i16)
                        n578 = Bundle("P3 2"="P3 2", "I3 2"="I3 2", "D3 2"="D3 2") -> (w1325:cluster{"P3 2":i16, "I3 2":i16, "D3 2":i16})  [unwired: 1 in]
                        n579 = Bundle("RF synth green feedback max"="RF synth green feedback max", i16 0) -> (w1317:cluster{"RF synth green feedback max":i16, i16})  [unwired: 1 in]
                        n580 = call "Slower PID.vi"("process variable"=w1313, "reset?"="Green FB Reset 2", "setpoint"="Green FB Setpoint 2", "PID gains (x 2^8)"=w1325, "output range"=w1317) -> ("output"=w1327:i16)  [unwired: 10 out]
                        n581 = To Unsigned Word Integer(number=w1327) -> (unsigned 16bit integer=w1326:u16)
                      }
                    }
                    n582 = feedback-in #48(w1304) -> ()
                  }
                  frame Enabled {
                  }
                }
              }
            }
            n583 = Split Number(x=w868) -> (hi(x)=w867:u32, lo(x)=w866:u32)
            n584 = Boolean To (0,1)(Boolean="+ phase (DIO)") -> (0, 1=w828:i16)
            n585 = Split Number(x=w867) -> (lo(x)=w865:u16)  [unwired: 1 out]
            n586 = Split Number(x=w866) -> (hi(x)=w864:u16, lo(x)=w863:u16)
            n587 = Split Number(x=w865) -> (hi(x)=w857:u8, lo(x)=w856:u8)
            n588 = Split Number(x=w864) -> (hi(x)=w855:u8, lo(x)=w854:u8)
            n589 = Split Number(x=w863) -> (hi(x)=w853:u8, lo(x)=w852:u8)
            n590 = Multiply(x=w828, y="Phase count adjustment (DIO)") -> (x*y=w824:i16)
            n591 = feedback #50(TRUE) -> (w813:bool)
            n592 = Not(x=w813) -> (.not. x?=w812:bool)
            n593 = feedback-in #50(w812) -> ()
            n594 = feedback #51(i16 0) -> (w826:i16)
            n595 = Subtract(x=w826, y=w824) -> (x-y=w825:i16)
            "DIO Relative phase" <- w825
            n596 = feedback-in #51(w825) -> ()
            n597 = Add(x=w831, y=w824) -> (x+y=w830:u32)
            n598 = Build Array "BD 1 nu Stack"(w857, w856, w855, w854, w853, w852) -> (w851:u8[])
            n599 = Not Equal?(x=w791, y=u8 3) -> (x != y?=w800:bool)
            n600 = case "Store in RF board F1 or F2" shown="True" w812 {
              tunnel: [w1023 w1027] -> w842
              tunnel: [u8 10 u8 4] -> w843
              tunnel: "Swap F1 and F2" -> [w1024 w1027]
              tunnel: "BD 2 Frequency 1" -> [_ w1026]
              tunnel: "BD 2 Frequency 2" -> [w1022 _]
              tunnel: [w1022 w1026] -> w808
              frame False {
                # "for RF synth controls\ngreen: F1/F2 stay same"
                # "F2 address (hex)"
                n601 = Not(x=w1024) -> (.not. x?=w1023:bool)
              }
              frame True {
                # "low chooses F1"
                # "F1 address (hex)"
              }
            }
            n602 = Select(t=w808, s="RF synth bd controls green", f=w807) -> (s? t:f=w806:u64)
            n603 = Split Number(x=w806) -> (hi(x)=w862:u32, lo(x)=w861:u32)
            n604 = Split Number(x=w862) -> (lo(x)=w860:u16)  [unwired: 1 out]
            n605 = Split Number(x=w861) -> (hi(x)=w859:u16, lo(x)=w858:u16)
            n606 = Split Number(x=w860) -> (hi(x)=w850:u8, lo(x)=w849:u8)
            n607 = Split Number(x=w859) -> (hi(x)=w848:u8, lo(x)=w847:u8)
            n608 = Split Number(x=w858) -> (hi(x)=w846:u8, lo(x)=w845:u8)
            n609 = feedback #52(u16 0 ("BD 2 Amplitude 3")) -> (w797:u16)
            n610 = Select(t=w797, s=w800, f=w799) -> (s? t:f=w798:u16)
            n611 = feedback-in #52(w798) -> ()
            n612 = And(x=w800, y=w803) -> (x .and. y?=w802:bool)
            n613 = Build Array "BD 2 nu Stack"(w850, w849, w848, w847, w846, w845) -> (w844:u8[])
            n614 = Select(t=w797, s=w802, f=w799) -> (s? t:f=w780:u16)
            n615 = flat-sequence "Update trap RF synth board settings to be used for the upcoming trap cycle." {
              tunnel: w844 -> [w971]
              tunnel: w851 -> [w972]
              tunnel: [w972] -> w795
              tunnel: [w971] -> w794
              tunnel: w843 -> [w973]
              tunnel: w795 -> [w975]
              tunnel: w794 -> [w974]
              tunnel: w782 -> [w986]
              tunnel: w784 -> [w985]
              tunnel: w783 -> [w984]
              frame #0 {
                # "To possibly delay\nthese writes to very\nend of loop (for x and\ny phase adjust)"
                n616 = call "Wait8"("Count(Ticks)"="Next trap write delay (ticks)") -> ()  [unwired: 1 out]
              }
              frame #1 {
                # "Next trap RF frequency:\n\nWrite next trap cycle frequency to buffer."
                n617 = for {
                  tunnel: w975 -> [w981] mode=indexing
                  tunnel: w974 -> [w980] mode=indexing
                  tunnel: w973 -> [w978]
                  i -> [w979]
                  n618 = To Unsigned Byte Integer(number=w979) -> (unsigned 8bit integer=w976:u8)
                  n619 = Add(x=w978, y=w976) -> (x+y=w977:u8)
                  n620 = call "write to RF synth bd.vi"("Address Byte"=w977, "BD 2 Byte"=w980, "BD 1 Byte"=w981) -> ()
                }
              }
              frame #2 {
                w982 = TRUE ("Connector1/DIO15")
                # "Send udclk high\n(BD 1 and 2) to make the new frequency active in F1 or F2 word. But it won't actually be the used frequency until FSK switches to it (begining of next cycle)."
                n621 = xnode "FPGA I/O Node"("Connector1/DIO30"=w982, "Connector1/DIO29"=w982) -> ()  [unwired: 2 in, 2 out]
              }
              frame #3 {
                w983 = FALSE ("Connector1/DIO15")
                n622 = xnode "FPGA I/O Node"("Connector1/DIO30"=w983, "Connector1/DIO29"=w983) -> ()  [unwired: 2 in, 2 out]
              }
              frame #4 {
                # "Next trap RF phase offset:\n\nSet the next trap cycle amplitude to the buffer. Won't become active until udclk is set high at proper time at the begining of the next cycle."
                n623 = case shown="True" w986 {
                  tunnel: w985 -> [_ w987]
                  tunnel: w984 -> [_ w988]
                  frame False {
                  }
                  frame True {
                    # "phase 1 address start"
                    n624 = for {
                      tunnel: w987 -> [w995] mode=indexing
                      tunnel: w988 -> [w994] mode=indexing
                      tunnel: u8 0 -> [w992]
                      i -> [w993]
                      n625 = To Unsigned Byte Integer(number=w993) -> (unsigned 8bit integer=w990:u8)
                      n626 = Add(x=w992, y=w990) -> (x+y=w991:u8)
                      n627 = call "write to RF synth bd.vi"("Address Byte"=w991, "BD 2 Byte"=w994, "BD 1 Byte"=w995) -> ()
                    }
                  }
                }
              }
              frame #5 {
                # "Prep to reset RF phase to zero at start of next cycle. Only reset BD 1. Do nothing to BD 2. This puts the settings in the buffer. A udclk high will make both this phase reset and possibly a new phase offset setting active."
                n628 = case shown="True" "RF phase reset before cycles" {
                  frame False {
                  }
                  frame True {
                    w998 = u8 66  # BD 1 reset
                    n629 = call "write to RF synth bd.vi"("Address Byte"=u8 31, "BD 2 Byte"=u8 2, "BD 1 Byte"=w998) -> ()
                  }
                }
              }
              frame #6 {
                # "Address"
                # "Data BD 2"
                # "Data BD 1"
                # "If phase reset wasn't chosen previously, these actions will have no affect. For both BD's, data should be binary 10, and address should be hex 1F (bin 01 1111)"
                # "This sets up the digital communication lines to restart phase accumulation (start RF running agin). It cancels out the possible phase reset. Just need to set WR DIO low then udclk DIOhigh  to make this happen. Doing this here early (and not using the usual board write function) speeds things up.\n\nRestarts RF (BD 1 only, BD2 never stopped in first place)."
                n630 = xnode "FPGA I/O Node"("Connector1/DIO0"=FALSE, "Connector1/DIO1"=FALSE, "Connector1/DIO2"=FALSE, "Connector1/DIO3"=FALSE, "Connector1/DIO4"=FALSE, "Connector1/DIO5"=FALSE, "Connector1/DIO6"=TRUE, "Connector1/DIO7"=FALSE, "Connector1/DIO8"=FALSE, "Connector1/DIO9"=TRUE, "Connector1/DIO10"=TRUE, "Connector1/DIO11"=TRUE, "Connector1/DIO12"=TRUE, "Connector1/DIO13"=TRUE, "Connector1/DIO20"=FALSE, "Connector1/DIO21"=FALSE, "Connector1/DIO22"=FALSE, "Connector1/DIO23"=FALSE, "Connector1/DIO24"=FALSE, "Connector1/DIO25"=FALSE, "Connector1/DIO26"=TRUE, "Connector1/DIO27"=FALSE) -> ()  [unwired: 22 in, 22 out]
              }
            }
            n631 = feedback #53(fxp<+,8,8> 0.0) -> (w777:fxp<+,8,8>)
            n632 = Increment(x=w777) -> (x+1=w775:fxp<+,8,8>)
            n633 = feedback-in #53(w775) -> ()
            n634 = case "Trap RF phase offset control methods" shown="3" "Phase offset method" {
              tunnel: [fxp<+,14,14> 0.0 ("Phase BD 1") w921 w936 w965] -> w785
              tunnel: "Phase Trap 1" -> [_ w922 w937 _]
              tunnel: w791 -> [_ w923 w938 w966]
              tunnel: [FALSE TRUE TRUE TRUE] -> w782
              tunnel: "Phase Trap 2" -> [_ w919 w934 _]
              tunnel: w775 -> [_ _ w933 _]
              frame 0, Default {
              }
              frame 1 {
                # "Constant increment of phase offset with each trap cycle. This results in a constant phase difference between trap cycles. \nOnly for traps 1 and 2 (set phase offset to zero for set three)."
                n635 = case shown="1, Default" w923 {
                  tunnel: w922 -> [_ _ w929]
                  tunnel: [w925 fxp<+,14,14> 0.0 w930] -> w921
                  tunnel: w919 -> [w924 _ _]
                  frame 2 {
                    n636 = feedback #54(fxp<+,14,14> 0.0) -> (w927:fxp<+,14,14>)
                    n637 = Add(x=w924, y=w927) -> (x+y=w925:fxp<+,14,14>)
                    n638 = feedback-in #54(w925) -> ()
                  }
                  frame 3 {
                  }
                  frame 1, Default {
                    n639 = feedback #55(fxp<+,14,14> 0.0) -> (w932:fxp<+,14,14>)
                    n640 = Add(x=w929, y=w932) -> (x+y=w930:fxp<+,14,14>)
                    n641 = feedback-in #55(w930) -> ()
                  }
                }
              }
              frame 2 {
                # "Changing increment of phase offset with each trap cycle. This results in a constant change in phase difference between trap cycles. \nOnly for traps 1 and 2 (set phase offset to zero for set three)."
                n642 = case shown="2" w938 {
                  tunnel: w937 -> [_ _ w948]
                  tunnel: [w939 fxp<+,14,14> 0.0 w946] -> w936
                  tunnel: w934 -> [w941 _ _]
                  tunnel: w933 -> [w942 _ w949]
                  frame 2 {
                    n643 = Multiply(x=w941, y=w942) -> (x*y=w940:fxp<+,16,16>)
                    n644 = feedback #56(fxp<+,14,14> 0.0) -> (w944:fxp<+,14,14>)
                    n645 = Add(x=w940, y=w944) -> (x+y=w939:fxp<+,14,14>)
                    n646 = feedback-in #56(w939) -> ()
                  }
                  frame 3 {
                  }
                  frame 1, Default {
                    n647 = Multiply(x=w948, y=w949) -> (x*y=w947:fxp<+,16,16>)
                    n648 = feedback #57(fxp<+,14,14> 0.0) -> (w951:fxp<+,14,14>)
                    n649 = Add(x=w947, y=w951) -> (x+y=w946:fxp<+,14,14>)
                    n650 = feedback-in #57(w946) -> ()
                  }
                }
              }
              frame 3 {
                w958 = u32 1013904223  # LCG constant C (add)
                w960 = fxp<+,21,21> 1664525.0  # LCG constant A (multiply)
                # "Set a random phase offset. Random number generated using the LCG method. Constants and method taken from NI white noise generator code (method is general though)."
                # "shift to 14 significant bits"
                n651 = feedback #58(u32 4294967295 ("seed")) -> (w955:u32)
                n652 = Multiply(x=w955, y=w960) -> (x*y=w959:u32)
                n653 = Split Number(x=w955) -> (hi(x)=w961:u16)  [unwired: 1 out]
                n654 = To Unsigned Word Integer(number=w961) -> (unsigned 16bit integer=w953:u16)
                n655 = Add(x=w959, y=w958) -> (x+y=w957:fxp<+,32,32>)
                n656 = To Unsigned Long Integer(number=w957) -> (unsigned 32bit integer=w954:u32)
                n657 = feedback-in #58(w954) -> ()
                n658 = Scale By Power Of 2(n=i8 -2 ("Uniform scale factor"), x=w953) -> (x*2^n=w962:u16)
                n659 = To Fixed-Point(number=w962) -> (fixed-point=w952:fxp<+,14,14>)  [unwired: 1 in]
                "Random phase generated" <- w952
                n660 = case shown="1, Default" w966 {
                  tunnel: [w967 fxp<+,14,14> 0.0 w969] -> w965
                  tunnel: w952 -> [w967 _ w969]
                  frame 2 {
                  }
                  frame 3 {
                  }
                  frame 1, Default {
                  }
                }
              }
            }
            n661 = To Unsigned Word Integer(number=w785) -> (unsigned 16bit integer=w790:u16)
            n662 = Split Number(x=w790) -> (hi(x)=w788:u8, lo(x)=w789:u8)
            n663 = Split Number(x=u16 0) -> (hi(x)=w786:u8, lo(x)=w787:u8)
            n664 = Build Array ("BD 1 A Stack")(w788, w789) -> (w784:u8[])
            n665 = Build Array ("BD 1 A Stack")(w786, w787) -> (w783:u8[])
          }
        }
      }
    }
  }
  n666 = while "532 nm green fluorescent laser interlacing (DO to IA 532 nm AOM ME amp)." {
    shift-right: [w1331] -> _
    shift-left: w2 -> [w1336]
    shift-right: [w1330] -> _
    shift-left: w3 -> [w1328]
    stop <- FALSE stop-if-true
    n667 = flat-sequence {
      tunnel: w1336 -> [w1339]
      tunnel: [w1338] -> w1334
      tunnel: [w1339] -> w1332
      tunnel: [w1340] -> w1329
      tunnel: w1328 -> [w1340]
      tunnel: [w1343] -> w1335
      tunnel: w1334 -> [w1343]
      tunnel: [w1342] -> w1333
      tunnel: w1332 -> [w1342]
      tunnel: w1329 -> [w1341]
      tunnel: [w1355] -> w1331
      tunnel: w1335 -> [w1374]
      tunnel: w1333 -> [w1371]
      tunnel: [w1344] -> w1330
      frame #0 {
        n668 = call "Loop Timer9"("Count(Ticks)"=w1339) -> ("Tick Count(Ticks)"=w1338:u32)
      }
      frame #1 {
        # "Then to PRL 440 amp\nOR to RF synth board FSK in"
        n669 = xnode "FPGA I/O Node"("Connector1/DIO37"=w1341, "Connector1/DIO38"=w1341, "Connector1/DIO39"=w1341, "Connector1/DIO26"=w1341, "Connector1/DIO27"=w1341, "Connector1/DIO32"=w1341) -> ()  [unwired: 6 in, 6 out]
      }
      frame #2 {
        n670 = feedback-in #59(w1374) -> ()
        n671 = feedback #59(w1374) -> (w1373:u32)
        n672 = Subtract(x=w1374, y=w1373) -> (x-y=w1372:u32)
        n673 = Subtract(x=w1372, y=w1371) -> (x-y=w1348:u32)
        n674 = Number To Boolean Array(number=w1348) -> (Boolean array=w1349:bool[])
        n675 = Or Array Elements(Boolean array=w1349) -> (logical OR=w1347:bool)
        n676 = Boolean To (0,1)(Boolean="+ phase (GI)") -> (0, 1=w1360:i16)
        n677 = Boolean To (0,1)(Boolean=w1347) -> (0, 1=w1354:i16)
        n678 = To Unsigned Byte Integer(number=w1354) -> (unsigned 8bit integer=w1351:u8)
        n679 = Multiply(x=w1360, y="Phase count adjustment (GI)") -> (x*y=w1357:i16)
        n680 = feedback #60(u8 0) -> (w1352:u8)
        n681 = Add(x=w1351, y=w1352) -> (x+y=w1350:u8)
        "GI Late Counter" <- w1350
        n682 = feedback-in #60(w1350) -> ()
        n683 = feedback #61(i16 0) -> (w1358:i16)
        n684 = Subtract(x=w1358, y=w1357) -> (x-y=w1356:i16)
        "GI Relative phase" <- w1356
        n685 = feedback-in #61(w1356) -> ()
        n686 = feedback #62(TRUE) -> (w1366:bool)
        n687 = case shown="2" "Operating Mode" {
          tunnel: [TRUE FALSE w1399] -> w1345
          tunnel: w1366 -> [_ _ w1396]
          frame 0, Default {
          }
          frame 1 {
          }
          frame 2 {
            n688 = Not(x=w1396) -> (.not. x?=w1398:bool)
            n689 = Select(t=w1398, s="Invert GI", f=w1396) -> (s? t:f=w1399:bool)
          }
        }
        n690 = Not(x=w1366) -> (.not. x?=w1363:bool)
        n691 = Select(t="Green interlace ON count", s=w1363, f="Green interlace OFF count") -> (s? t:f=w1368:u16)
        n692 = Subtract(x=w1368, y=w1348) -> (x-y=w1361:u32)
        n693 = Add(x=w1361, y=w1357) -> (x+y=w1355:u32)
        n694 = feedback-in #62(w1363) -> ()
        n695 = case shown="True" "Green long-scale interlacing" {
          tunnel: w1345 -> [w1375 w1383]
          tunnel: [w1375 w1384] -> w1344
          frame False {
          }
          frame True {
            n696 = feedback #63(i16 1) -> (w1390:i16)
            n697 = Increment(x=w1390) -> (x+1=w1389:i16)
            n698 = feedback #64("Number of ON cycles") -> (w1376:i16)
            n699 = Greater?(x=w1376, y=w1390) -> (0:w1385:bool)
            n700 = Select(t=w1389, s=w1385, f=i16 1) -> (s? t:f=w1387:i16)
            n701 = feedback-in #63(w1387) -> ()
            n702 = feedback #65(TRUE) -> (w1382:bool)
            n703 = Not(x=w1382) -> (.not. x?=w1381:bool)
            n704 = Select(t=w1382, s=w1385, f=w1381) -> (s? t:f=w1380:bool)
            n705 = Select(t="Number of ON cycles", s=w1380, f="Number of OFF cycles") -> (s? t:f=w1378:i16)
            n706 = feedback-in #64(w1378) -> ()
            n707 = feedback-in #65(w1380) -> ()
            n708 = case shown="False" w1380 {
              tunnel: [FALSE w1393] -> w1384
              tunnel: w1383 -> [_ w1393]
              frame False {
              }
              frame True {
              }
            }
          }
        }
      }
    }
  }
  n709 = while "Green excitation laser feedback measurement" {
    shift-right: [w1400] -> _
    shift-left: w2 -> [w1405]
    stop <- FALSE stop-if-true
    n710 = flat-sequence {
      tunnel: w1405 -> [w1407]
      tunnel: [w1408] -> w1403
      tunnel: [w1407] -> w1401
      tunnel: [w1415] -> w1404
      tunnel: w1403 -> [w1415]
      tunnel: [w1414] -> w1402
      tunnel: w1401 -> [w1414]
      tunnel: [w1427] -> w1400
      tunnel: w1404 -> [w1438]
      tunnel: w1402 -> [w1435]
      frame #0 {
        n711 = call "Loop Timer6"("Count(Ticks)"=w1407) -> ("Tick Count(Ticks)"=w1408:u32)
      }
      frame #1 {
        n712 = xnode "FPGA I/O Node"("Connector1/DIO35"=TRUE) -> ("Chassis2/Mod2/AI0"=w1413:i16, "Chassis2/Mod2/AI1"=w1412:i16, "Chassis2/Mod2/AI2"=w1409:i16)  [unwired: 4 in, 4 out]
        "Green FB Sum" <- w1409
        n713 = Bundle("Chassis2/Mod2/AI0"=w1413, "Chassis2/Mod2/AI1"=w1412, "Chassis2/Mod2/AI2"=w1409) -> (→"Green FB Signals":T10)  [unwired: 1 out]
      }
      frame #2 {
        n714 = feedback-in #66(w1438) -> ()
        n715 = feedback #66(w1438) -> (w1437:u32)
        n716 = Subtract(x=w1438, y=w1437) -> (x-y=w1436:u32)
        n717 = xnode "FPGA I/O Node"("Connector1/DIO35"=FALSE) -> ()  [unwired: 1 in, 1 out]
        n718 = Subtract(x=w1436, y=w1435) -> (x-y=w1417:u32)
        n719 = Subtract(x="Green FB Count", y=w1417) -> (x-y=w1431:u32)
        n720 = Number To Boolean Array(number=w1417) -> (Boolean array=w1418:bool[])
        n721 = Or Array Elements(Boolean array=w1418) -> (logical OR=w1416:bool)
        "Green FB Late?" <- w1416
        n722 = Boolean To (0,1)(Boolean="+ phase (Green FB)") -> (0, 1=w1429:i16)
        n723 = Boolean To (0,1)(Boolean=w1416) -> (0, 1=w1423:i16)
        n724 = Multiply(x=w1429, y="Phase count adjustment (Green FB)") -> (x*y=w1424:i16)
        n725 = Add(x=w1431, y=w1424) -> (x+y=w1427:u32)
        n726 = To Unsigned Word Integer(number=w1423) -> (unsigned 16bit integer=w1420:u16)
        n727 = feedback #67(i16 0) -> (w1426:i16)
        n728 = Subtract(x=w1426, y=w1424) -> (x-y=w1425:i16)
        "Green FB Relative Phase" <- w1425
        n729 = feedback-in #67(w1425) -> ()
        n730 = feedback #68(u16 0) -> (w1421:u16)
        n731 = Add(x=w1420, y=w1421) -> (x+y=w1419:u16)
        "Green Late Counter" <- w1419
        n732 = feedback-in #68(w1419) -> ()
      }
    }
  }
  n733 = while "Control APD data integration - stream to host" {
    shift-right: [w1441] -> _
    shift-left: w5 -> [w1446]
    stop <- FALSE stop-if-true
    n734 = flat-sequence {
      tunnel: w1446 -> [w1448]
      tunnel: [w1449] -> w1444
      tunnel: [w1448] -> w1442
      tunnel: [w1457] -> w1445
      tunnel: w1444 -> [w1457]
      tunnel: [w1456] -> w1443
      tunnel: w1442 -> [w1456]
      tunnel: [w1455] -> w1440
      tunnel: [w1454] -> w1439
      tunnel: [w1491] -> w1441
      tunnel: w1445 -> [w1503]
      tunnel: w1443 -> [w1500]
      tunnel: w1440 -> [w1484]
      tunnel: w1439 -> [w1483]
      frame #0 {
        n735 = call "Loop Timer4"("Count(Ticks)"=w1448) -> ("Tick Count(Ticks)"=w1449:u32)
      }
      frame #1 {
        n736 = flat-sequence {
          tunnel: [w1459] -> w1453
          tunnel: w1453 -> [w1461]
          tunnel: [w1463] -> w1452
          tunnel: [w1462] -> w1451
          tunnel: [w1461] -> w1450
          tunnel: [w1469] -> w1454
          tunnel: [w1470] -> w1455
          tunnel: w1452 -> [w1470]
          tunnel: w1451 -> [w1469]
          tunnel: w1450 -> [w1468]
          frame #0 {
            # "use two separate variable so each APD won't\nhave to wait to read"
            n737 = feedback #69(FALSE) -> (w1458:bool)
            "APD1 out state" <- w1458
            "APD2 out state" <- w1458
            n738 = Not(x=w1458) -> (.not. x?=w1459:bool)
            n739 = feedback-in #69(w1459) -> ()
          }
          frame #1 {
            n740 = local read "APD 1 Counts 1"() -> (w1467:u32)
            n741 = local read "APD 1 Counts 0"() -> (w1466:u32)
            n742 = local read "APD 2 Counts 1"() -> (w1465:u32)
            n743 = local read "APD 2 Counts 0"() -> (w1464:u32)
            n744 = Select(t=w1467, s=w1461, f=w1466) -> (s? t:f=w1463:u32)
            n745 = Select(t=w1465, s=w1461, f=w1464) -> (s? t:f=w1462:u32)
          }
          frame #2 {
            n746 = case shown="True" w1468 {
              frame False {
                w1471 = u32 0 ("APD 1 Counts 0")
                n747 = local write "APD 1 Counts 0"(w1471) -> ()
                n748 = local write "APD 2 Counts 0"(w1471) -> ()
              }
              frame True {
                w1472 = u32 0 ("APD 1 Counts 1")
                n749 = local write "APD 1 Counts 1"(w1472) -> ()
                n750 = local write "APD 2 Counts 1"(w1472) -> ()
              }
            }
          }
        }
      }
      frame #2 {
        n751 = feedback-in #70(w1503) -> ()
        n752 = feedback #70(w1503) -> (w1502:u32)
        n753 = Subtract(x=w1503, y=w1502) -> (x-y=w1501:u32)
        n754 = Subtract(x=w1501, y=w1500) -> (x-y=w1476:u32)
        n755 = case shown="True" "APD to FIFO" {
          tunnel: w1484 -> [_ w1506]
          tunnel: w1483 -> [_ w1504]
          frame False {
          }
          frame True {
            n756 = flat-sequence {
              tunnel: 0 ("Timeout") -> [w1508]
              tunnel: w1506 -> [w1509]
              tunnel: [w1508] -> w1505
              tunnel: w1505 -> [w1511]
              tunnel: w1504 -> [w1510]
              frame #0 {
                n757 = xnode ("FIFO Write")("Element"=w1509, "Timeout"=w1508) -> ()  [unwired: 1 in, 2 out]
              }
              frame #1 {
                n758 = xnode ("FIFO Write")("Element"=w1510, "Timeout"=w1511) -> ()  [unwired: 1 in, 2 out]
              }
            }
          }
        }
        n759 = Subtract(x="APD Acq Rate Count", y=w1476) -> (x-y=w1492:u32)
        n760 = Number To Boolean Array(number=w1476) -> (Boolean array=w1477:bool[])
        n761 = Or Array Elements(Boolean array=w1477) -> (logical OR=w1475:bool)
        "APD Acq Late?" <- w1475
        n762 = Boolean To (0,1)(Boolean=w1475) -> (0, 1=w1482:i16)
        n763 = To Unsigned Word Integer(number=w1482) -> (unsigned 16bit integer=w1479:u16)
        n764 = Boolean To (0,1)(Boolean="+ phase (APD Acq)") -> (0, 1=w1488:i16)
        n765 = feedback #71(u16 0) -> (w1480:u16)
        n766 = Add(x=w1479, y=w1480) -> (x+y=w1478:u16)
        "APD Acq Late Counter" <- w1478
        n767 = feedback-in #71(w1478) -> ()
        n768 = Multiply(x=w1488, y="Phase Count Adjustment (APD Acq)") -> (x*y=w1485:i16)
        n769 = Add(x=w1492, y=w1485) -> (x+y=w1491:u32)
        n770 = feedback #72(i16 0) -> (w1490:i16)
        n771 = Subtract(x=w1490, y=w1485) -> (x-y=w1487:i16)
        "APD Acq Relative Phase" <- w1487
        n772 = feedback-in #72(w1487) -> ()
        n773 = To Word Integer(number=w1484) -> (16bit integer=w1493:i16)
        n774 = To Word Integer(number=w1483) -> (16bit integer=w1494:i16)
        n775 = Multiply(x="APD 1 AO scale factor", y=w1493) -> (x*y=w1474:i16)
        n776 = Multiply(x="APD 2 AO scale factor", y=w1494) -> (x*y=w1473:i16)
        n777 = xnode "FPGA I/O Node"("Connector0/AO6"=w1474, "Connector0/AO7"=w1473) -> ()  [unwired: 2 in, 2 out]
      }
    }
  }
  n778 = disable-structure shown="Disabled" {
    disable-tunnel: w2 -> [w1512 _]
    frame Disabled {
      n779 = while "APD 3 Counter" {
        tunnel: w1512 -> [_]
        stop <- FALSE stop-if-true
        n780 = flat-sequence {
          frame #0 {
            n781 = xnode "FPGA I/O Method Node"("FPGA I/O In"=refnum<k21> "Connector0/DIO12" ("APD 2 DO"), "Timeout"=-1) -> ()  [unwired: 2 out]
          }
          frame #1 {
            n782 = local read "APD3 int gate"() -> (w1516:bool)
            n783 = case shown="True" w1516 {
              frame False {
              }
              frame True {
                n784 = local read item#-1() -> (w1517)
                n785 = case shown="True" w1517 {
                  frame False {
                    n786 = local read "APD 3 Counts 0"() -> (w1519:u32)
                    n787 = Increment(x=w1519) -> (x+1=→"APD 3 Counts 0":u32)
                  }
                  frame True {
                    n788 = local read "APD 3 Counts 1"() -> (w1521:u32)
                    n789 = Increment(x=w1521) -> (x+1=→"APD 3 Counts 1":u32)
                  }
                }
              }
            }
          }
        }
      }
    }
    frame Enabled {
    }
  }
  n790 = disable-structure shown="Disabled" {
    disable-tunnel: w2 -> [w1523 _]
    disable-tunnel: w4 -> [w1522 _]
    frame Disabled {
      n791 = while "APD 3 Gating" {
        shift-right: [w1527] -> _
        shift-left: w1523 -> [w1532]
        shift-right: [w1526] -> _
        shift-left: w1522 -> [w1524]
        stop <- FALSE stop-if-true
        n792 = flat-sequence {
          tunnel: w1532 -> [w1535]
          tunnel: [w1534] -> w1530
          tunnel: [w1535] -> w1528
          tunnel: [w1536] -> w1525
          tunnel: w1524 -> [w1536]
          tunnel: [w1539] -> w1531
          tunnel: w1530 -> [w1539]
          tunnel: [w1538] -> w1529
          tunnel: w1528 -> [w1538]
          tunnel: w1525 -> [w1537]
          tunnel: [w1560] -> w1527
          tunnel: w1531 -> [w1571]
          tunnel: w1529 -> [w1568]
          tunnel: [w1540] -> w1526
          frame #0 {
            n793 = call "Loop Timer5"("Count(Ticks)"=w1535) -> ("Tick Count(Ticks)"=w1534:u32)
          }
          frame #1 {
            # "Signal maybe then sent through \na transistor before APD"
            n794 = xnode "FPGA I/O Node"("Connector0/DIO2"=w1537) -> ()  [unwired: 1 in, 1 out]
            "APD3 int gate" <- w1537
          }
          frame #2 {
            n795 = local read "APD Gate OFF Count"() -> (w1545:u16)
            n796 = local read "APD Gate ON Count"() -> (w1546:u16)
            n797 = feedback #73(TRUE) -> (w1565:bool)
            n798 = feedback-in #74(w1571) -> ()
            n799 = feedback #74(w1571) -> (w1570:u32)
            n800 = Not(x=w1565) -> (.not. x?=w1563:bool)
            n801 = feedback-in #73(w1563) -> ()
            n802 = Subtract(x=w1571, y=w1570) -> (x-y=w1569:u32)
            n803 = Select(t=w1546, s=w1563, f=w1545) -> (s? t:f=w1567:u16)
            n804 = Subtract(x=w1569, y=w1568) -> (x-y=w1548:u32)
            n805 = Subtract(x=w1567, y=w1548) -> (x-y=w1559:u32)
            n806 = Number To Boolean Array(number=w1548) -> (Boolean array=w1549:bool[])
            n807 = Or Array Elements(Boolean array=w1549) -> (logical OR=w1547:bool)
            n808 = Boolean To (0,1)(Boolean=w1547) -> (0, 1=w1554:i16)
            n809 = Boolean To (0,1)(Boolean="+ phase (APD 3 Gate)") -> (0, 1=w1557:i16)
            n810 = To Unsigned Byte Integer(number=w1554) -> (unsigned 8bit integer=w1551:u8)
            n811 = Multiply(x=w1557, y="Phase count adjustment (APD 3 Gate)") -> (x*y=w1555:i16)
            n812 = feedback #75(u8 0) -> (w1552:u8)
            n813 = Add(x=w1551, y=w1552) -> (x+y=w1550:u8)
            "APD 3 Gate Late Counter" <- w1550
            n814 = feedback-in #75(w1550) -> ()
            n815 = Add(x=w1559, y=w1555) -> (x+y=w1560:u32)
            n816 = feedback #76(i16 0) -> (w1562:i16)
            n817 = Subtract(x=w1562, y=w1555) -> (x-y=w1561:i16)
            "APD 3 Gate Relative Phase" <- w1561
            n818 = feedback-in #76(w1561) -> ()
            n819 = local read "APD Gate Operating Mode"() -> (w1544:u8)
            n820 = case shown="2" w1544 {
              tunnel: [TRUE FALSE w1574] -> w1541
              tunnel: w1565 -> [_ _ w1574]
              frame 0, Default {
              }
              frame 1 {
              }
              frame 2 {
              }
            }
            n821 = local read "Invert APD Gate"() -> (w1543:bool)
            n822 = Not(x=w1541) -> (.not. x?=w1542:bool)
            n823 = Select(t=w1542, s=w1543, f=w1541) -> (s? t:f=w1540:bool)
          }
        }
      }
    }
    frame Enabled {
    }
  }
  n824 = disable-structure shown="Disabled" {
    disable-tunnel: w2 -> [w1577 _]
    disable-tunnel: w3 -> [w1576 _]
    frame Disabled {
      n825 = while "633 nm red  fluorescent laser interlacing (DO to IA 633 nm AOM ME amp)." {
        shift-right: [w1698] -> _
        shift-left: w1577 -> [w1703]
        shift-right: [w1697] -> _
        shift-left: w1576 -> [w1695]
        stop <- FALSE stop-if-true
        n826 = flat-sequence {
          tunnel: w1703 -> [w1706]
          tunnel: [w1705] -> w1701
          tunnel: [w1706] -> w1699
          tunnel: [w1707] -> w1696
          tunnel: w1695 -> [w1707]
          tunnel: [w1710] -> w1702
          tunnel: w1701 -> [w1710]
          tunnel: [w1709] -> w1700
          tunnel: w1699 -> [w1709]
          tunnel: w1696 -> [w1708]
          tunnel: [w1719] -> w1698
          tunnel: w1702 -> [w1739]
          tunnel: w1700 -> [w1736]
          tunnel: [w1728] -> w1697
          frame #0 {
            n827 = call "Loop Timer8"("Count(Ticks)"=w1706) -> ("Tick Count(Ticks)"=w1705:u32)
          }
          frame #1 {
            # "Then to PRL 440 amp"
            n828 = xnode "FPGA I/O Node"("Connector1/DIO32"=w1708) -> ()  [unwired: 1 in, 1 out]
          }
          frame #2 {
            n829 = feedback-in #77(w1739) -> ()
            n830 = feedback #77(w1739) -> (w1738:u32)
            n831 = Subtract(x=w1739, y=w1738) -> (x-y=w1737:u32)
            n832 = Subtract(x=w1737, y=w1736) -> (x-y=w1712:u32)
            n833 = Number To Boolean Array(number=w1712) -> (Boolean array=w1713:bool[])
            n834 = Or Array Elements(Boolean array=w1713) -> (logical OR=w1711:bool)
            n835 = Boolean To (0,1)(Boolean="+ phase (RI)") -> (0, 1=w1724:i16)
            n836 = Multiply(x=w1724, y="Phase count adjustment (RI)") -> (x*y=w1721:i16)
            n837 = Boolean To (0,1)(Boolean=w1711) -> (0, 1=w1718:i16)
            n838 = To Unsigned Byte Integer(number=w1718) -> (unsigned 8bit integer=w1715:u8)
            n839 = feedback #78(i16 0) -> (w1722:i16)
            n840 = feedback #79(u8 0) -> (w1716:u8)
            n841 = Add(x=w1715, y=w1716) -> (x+y=w1714:u8)
            "RI Late Counter" <- w1714
            n842 = feedback-in #79(w1714) -> ()
            n843 = Subtract(x=w1722, y=w1721) -> (x-y=w1720:i16)
            "RI Relative phase" <- w1720
            n844 = feedback-in #78(w1720) -> ()
            n845 = feedback #80(TRUE) -> (w1731:bool)
            n846 = case shown="2" "Red Laser Operating Mode" {
              tunnel: [TRUE FALSE w1745] -> w1728
              tunnel: w1731 -> [_ _ w1742]
              frame 0, Default {
              }
              frame 1 {
              }
              frame 2 {
                n847 = Not(x=w1742) -> (.not. x?=w1744:bool)
                n848 = Select(t=w1744, s="Invert RI", f=w1742) -> (s? t:f=w1745:bool)
              }
            }
            n849 = Not(x=w1731) -> (.not. x?=w1727:bool)
            n850 = Select(t="Red interlace ON count", s=w1727, f="Red interlace OFF count") -> (s? t:f=w1733:u16)
            n851 = Subtract(x=w1733, y=w1712) -> (x-y=w1725:u32)
            n852 = Add(x=w1725, y=w1721) -> (x+y=w1719:u32)
            n853 = feedback-in #80(w1727) -> ()
          }
        }
      }
      n854 = while "473 nm blue  fluorescent laser interlacing (DO to blue laser digital control input)." {
        shift-right: [w1594] -> _
        shift-left: w1577 -> [w1597]
        shift-right: [w1593] -> _
        shift-left: w1576 -> [w1591]
        shift-right: [w1586] -> _
        shift-left: _ -> [w1585]
        shift-right: [w1578] -> _
        shift-left: u16 0 -> [w1581]
        stop <- FALSE stop-if-true
        n855 = flat-sequence {
          tunnel: w1597 -> [w1600]
          tunnel: [w1599] -> w1596
          tunnel: [w1600] -> w1595
          tunnel: [w1603] -> w1592
          tunnel: w1591 -> [w1603]
          tunnel: w1585 -> [w1602]
          tunnel: [w1602] -> w1584
          tunnel: [w1601] -> w1582
          tunnel: w1581 -> [w1601]
          tunnel: [w1608] -> w1590
          tunnel: w1596 -> [w1608]
          tunnel: [w1607] -> w1589
          tunnel: w1595 -> [w1607]
          tunnel: w1592 -> [w1606]
          tunnel: w1584 -> [w1605]
          tunnel: [w1605] -> w1583
          tunnel: w1582 -> [w1604]
          tunnel: [w1604] -> w1580
          tunnel: [w1613] -> w1588
          tunnel: [w1612] -> w1587
          tunnel: w1589 -> [w1612]
          tunnel: w1590 -> [w1613]
          tunnel: w1583 -> [w1611]
          tunnel: w1580 -> [w1610]
          tunnel: [w1609] -> w1579
          tunnel: [w1670] -> w1594
          tunnel: w1588 -> [w1688]
          tunnel: w1587 -> [w1685]
          tunnel: [w1658] -> w1593
          tunnel: [w1656] -> w1586
          tunnel: w1579 -> [w1653]
          tunnel: [w1654] -> w1578
          frame #0 {
            n856 = call "Loop Timer7"("Count(Ticks)"=w1600) -> ("Tick Count(Ticks)"=w1599:u32)
          }
          frame #1 {
            n857 = xnode "FPGA I/O Node"("Connector1/DIO28"=w1606) -> ()  [unwired: 1 in, 1 out]
          }
          frame #2 {
            n858 = case shown="True" w1611 {
              tunnel: w1610 -> [w1614 w1616]
              tunnel: [w1614 w1615] -> w1609
              frame False {
              }
              frame True {
                n859 = flat-sequence {
                  tunnel: [w1622] -> w1619
                  tunnel: [w1621] -> w1618
                  tunnel: [w1620] -> w1617
                  tunnel: w1616 -> [w1620]
                  tunnel: w1619 -> [w1639]
                  tunnel: w1618 -> [w1636]
                  tunnel: w1617 -> [w1638]
                  tunnel: [w1637] -> w1615
                  frame #0 {
                    # "5 ns timing resolution"
                    n860 = node-c288() -> (w1625:T7)  [unwired: 1 in]
                    n861 = timed-loop {
                      timing: w1625 -> [_]
                      timing-out: [_] -> w1624
                      tunnel: "Lifetime timeout APD1" -> [w1631]
                      tunnel: [w1626] -> w1621
                      tunnel: [w1627] -> w1622
                      i -> [w1628]
                      stop <- w1630 stop-if-true
                      n862 = xnode "FPGA I/O Node"() -> ("Connector0/DIO5"=w1629:bool)  [unwired: 1 in, 1 out]
                      n863 = To Unsigned Word Integer(number=w1628) -> (unsigned 16bit integer=w1626:u16)
                      n864 = Equal?(x=w1631, y=w1626) -> (x = y?=w1627:bool)
                      n865 = Or(x=w1629, y=w1627) -> (x .or. y?=w1630:bool)
                    }
                    n866 = node-c288(w1624) -> ()
                  }
                  frame #1 {
                    n867 = Not(x=w1639) -> (.not. x?=w1640:bool)
                    n868 = case shown="True" w1640 {
                      tunnel: w1636 -> [_ w1642]
                      tunnel: w1638 -> [w1641 w1644]
                      tunnel: [w1641 w1643] -> w1637
                      frame False {
                        # "timed out, do nothing"
                      }
                      frame True {
                        # "photon detected,record time"
                        n869 = case shown="True" "Lifetime to FIFO" {
                          tunnel: w1642 -> [_ w1650]
                          tunnel: w1644 -> [w1646 w1648]
                          tunnel: [w1646 w1647] -> w1643
                          frame False {
                            # "don't record time\n(can't if doing force feedback)"
                          }
                          frame True {
                            # "number of events in fifo"
                            n870 = xnode ("FIFO Method Node")("Element"=w1650, "Timeout"=0) -> ()  [unwired: 1 in, 2 out]
                            n871 = Increment(x=w1648) -> (x+1=w1647:u16)
                          }
                        }
                        "lifetime (ticks)" <- w1642
                      }
                    }
                  }
                }
              }
            }
          }
          frame #3 {
            # "Reading fifo is tricky here since\nunknown # of events"
            # "For lifetime measurement:\nInterlacing and pulse falling"
            n872 = feedback-in #81(w1688) -> ()
            n873 = feedback #81(w1688) -> (w1687:u32)
            n874 = Subtract(x=w1688, y=w1687) -> (x-y=w1686:u32)
            n875 = Subtract(x=w1686, y=w1685) -> (x-y=w1663:u32)
            n876 = Number To Boolean Array(number=w1663) -> (Boolean array=w1664:bool[])
            n877 = Or Array Elements(Boolean array=w1664) -> (logical OR=w1662:bool)
            n878 = Boolean To (0,1)(Boolean="+ phase (BI D)") -> (0, 1=w1675:i16)
            n879 = Multiply(x=w1675, y="Phase count adjustment (BI D)") -> (x*y=w1672:i16)
            n880 = Boolean To (0,1)(Boolean=w1662) -> (0, 1=w1669:i16)
            n881 = To Unsigned Byte Integer(number=w1669) -> (unsigned 8bit integer=w1666:u8)
            n882 = feedback #82(i16 0) -> (w1673:i16)
            n883 = feedback #83(u8 0) -> (w1667:u8)
            n884 = Add(x=w1666, y=w1667) -> (x+y=w1665:u8)
            "Blue Late Counter (D)" <- w1665
            n885 = feedback-in #83(w1665) -> ()
            n886 = Subtract(x=w1673, y=w1672) -> (x-y=w1671:i16)
            "BI Relative phase (D)" <- w1671
            n887 = feedback-in #82(w1671) -> ()
            n888 = feedback #84(TRUE) -> (w1680:bool)
            n889 = case shown="2" "Blue Laser Operating Mode (D)" {
              tunnel: [TRUE FALSE w1694] -> w1658
              tunnel: w1680 -> [_ _ w1691]
              frame 0, Default {
              }
              frame 1 {
              }
              frame 2 {
                n890 = Not(x=w1691) -> (.not. x?=w1693:bool)
                n891 = Select(t=w1693, s="Invert BI (D)", f=w1691) -> (s? t:f=w1694:bool)
              }
            }
            n892 = Subtract(x=w1653, y="Lifetime events to read blue") -> (x-y=w1651:u16)
            n893 = Not(x=w1680) -> (.not. x?=w1678:bool)
            n894 = Select(t="Blue interlace ON count (D)", s=w1678, f="Blue interlace OFF count (D)") -> (s? t:f=w1682:u16)
            n895 = Subtract(x=w1682, y=w1663) -> (x-y=w1676:u32)
            n896 = Add(x=w1676, y=w1672) -> (x+y=w1670:u32)
            n897 = feedback-in #84(w1678) -> ()
            n898 = Select(t=w1651, s="Lifetime read blue fifo", f=w1653) -> (s? t:f=w1654:u16)
            "lifetime events in fifo" <- w1654
            n899 = Equal?(x="Blue Laser Operating Mode (D)", y=u8 2) -> (x = y?=w1659:bool)
            n900 = Not(x=w1658) -> (.not. x?=w1657:bool)
            n901 = And(x=w1657, y=w1659) -> (x .and. y?=w1656:bool)
          }
        }
      }
    }
    frame Enabled {
    }
  }
